vi "Strategy 5_Autotuning PID_With GUI_Modified for Testing - Copy.vi"() -> ()   [LabVIEW 2018]
doc: "This example demonstrates how to use the PID Design function to obtain PID parameters based on measured process."
uses:
  <vilib>/DAQmx/write.llb/DAQmx Write (Digital 1D Bool 1Chan 1Samp).vi
  <vilib>/DAQmx/read.llb/DAQmx Read (Analog 1D DBL NChan 1Samp).vi
  <vilib>/Instr/_visa.llb/VISA Configure Serial Port (Instr).vi
  <vilib>/DAQmx/create/channels.llb/DAQmx Create Channel (DO-Digital Output).vi
  <vilib>/DAQmx/miscellaneous.llb/DAQmx Fill In Error Info.vi
  <vilib>/addons/control/pid/pid.llb/PID Advanced (DBL).vi
  <vilib>/addons/control/pid/autopid.llb/PID Autotuning Design (Ziegler-Nichols).vi
  <vilib>/addons/control/pid/autopid.llb/PID Autotuning Design (Cohen-Coon).vi
  <vilib>/addons/control/pid/autopid.llb/PID Autotuning Design (Chien-Hrones-Reswick).vi
  <vilib>/addons/control/pid/autopid.llb/PID Autotuning Design (Internal Model Control).vi
  <vilib>/addons/control/pid/NI_PID_autopid.lvlib
  <vilib>/addons/control/pid/NI_PID_pid.lvlib
  <vilib>/ptbypt/NI_PtbyPt.lvlib
panel:
  out "Tracker 4 - X,Y,Z":cluster{"x":sgl, "y":sgl, "z":sgl}(graph)
  out "Tracker 3 - X,Y,Z":cluster{"x":sgl, "y":sgl, "z":sgl}(graph)
  out "Tracker 2 - X,Y,Z":cluster{"x":sgl, "y":sgl, "z":sgl}(graph)
  out "Tracker 1 - X,Y,Z":cluster{"x":sgl, "y":sgl, "z":sgl}(graph)
  in  "Set Point 1,5":dbl
  out "Real time Data 1,5":dbl[][](graph)
  in  "Set Point 3,4":dbl
  out "Real time Data 3,4":dbl[][](graph)
  in  "Set Point 2":dbl
  out "Real time Data 2":dbl[][](graph)
  in  "Set Point 7":dbl
  out "Real time Data 7":dbl[][](graph)
  in  "Set Point  6,8,9,10":dbl
  out "Real time Data 6,8,9,10":dbl[][](graph)
  in  "Set Point 11,12":dbl
  out "Real time Data -11,12":dbl[][](graph)
  out "error out":errorcluster {"code" format="%.0x"}
  in  "XYZAER":T1(array[cluster]) {"r" format="%1_6f"; "e" format="%1_6f"; "a" format="%1_6f"; "z" format="%1_6f"; "y" format="%1_6f"; "x" format="%1_6f"}
  out "Start Time Text":string
  out "Stop Time Text":string
  out "Elapsed Time Text":string
  out "HostFrameCount":u32
  out "Loop Iter":i32
  out "PnoData":bool
  in  "stop":bool
  out "?":bool
  in  "Muscle Control":T2(tab)=enum."M-11,12"
  out "Tuned PID gains 12":T3={"proportional gain (Kc)"=1.9838195929127882, "integral time (Ti, min)"=0.01995856284686879, "derivative time (Td, min)"=0.0} {"derivative time (Td, min)" format="%#.6g"; "integral time (Ti, min)" format="%#.6g"; "proportional gain (Kc)" format="%#.6g"}
  in  "Accept gain 12":bool
  in  "Control 12":T4(tab)
  in  "Ziegler-Nichols speed 12":u16(ring) items=["Fast", "Normal", "Slow"]
  in  "Tuning specifications 12":u16(ring) items=["Regulator - 0 %", "Regulator -  20%", "Servo - 0%", "Servo - 20%"]
  in  "Multiplicative factor 12":dbl(slide)=1.0 scale=0.01..100.0
  in  "Type of controller 12":u16(ring)=2 items=["P", "PI", "PID"]
  in  "Stop 12":bool
  in  "PID Gains 12":T3={"proportional gain (Kc)"=0.1625, "integral time (Ti, min)"=1.25, "derivative time (Td, min)"=0.0} {"derivative time (Td, min)" format="%#.6g"; "integral time (Ti, min)" format="%#.6g"; "proportional gain (Kc)" format="%#.6g"}
  in  "Autotune 12":bool
  in  "Reinitialize 12":bool
  in  "Excitation 12":dbl=0.5 format="%.2f"
  in  "Automatic 12":bool=TRUE
  in  "MV: 12":dbl(slide)=20.39115328927357 scale=-100.0..100.0
  out "PWM Output 12":bool
  in  "Median sample length 21":i32=100
  in  "INLET 1,5 ON/OFF 3":bool=TRUE
  out "Tuned PID gains 9":T3={"proportional gain (Kc)"=1.9838195929127882, "integral time (Ti, min)"=0.01995856284686879, "derivative time (Td, min)"=0.0} {"derivative time (Td, min)" format="%#.6g"; "integral time (Ti, min)" format="%#.6g"; "proportional gain (Kc)" format="%#.6g"}
  in  "Accept gain 9":bool
  in  "Type of controller 9":u16(ring)=2 items=["P", "PI", "PID"]
  in  "Excitation 9":dbl=0.5 format="%.2f"
  in  "Control 9":T4(tab)
  in  "Ziegler-Nichols speed 9":u16(ring) items=["Fast", "Normal", "Slow"]
  in  "Tuning specifications 9":u16(ring) items=["Regulator - 0 %", "Regulator -  20%", "Servo - 0%", "Servo - 20%"]
  in  "Multiplicative factor 9":dbl(slide)=1.0 scale=0.01..100.0
  in  "Stop 9":bool
  in  "PID Gains 9":T3={"proportional gain (Kc)"=0.1625, "integral time (Ti, min)"=1.25, "derivative time (Td, min)"=0.0} {"derivative time (Td, min)" format="%#.6g"; "integral time (Ti, min)" format="%#.6g"; "proportional gain (Kc)" format="%#.6g"}
  in  "Autotune 9":bool
  in  "Reinitialize 9":bool
  in  "Automatic 9":bool=TRUE
  in  "MV: 9":dbl(slide)=20.39115328927357 scale=-100.0..100.0
  out "PWM Output 9":bool
  in  "Median sample length 18":i32=100
  in  "INLET 3,4 ON/OFF 2":bool=TRUE
  out "Tuned PID gains 8":T3={"proportional gain (Kc)"=1.9838195929127882, "integral time (Ti, min)"=0.01995856284686879, "derivative time (Td, min)"=0.0} {"derivative time (Td, min)" format="%#.6g"; "integral time (Ti, min)" format="%#.6g"; "proportional gain (Kc)" format="%#.6g"}
  in  "Accept gain 8":bool
  in  "Control 8":T4(tab)
  in  "Ziegler-Nichols speed 8":u16(ring) items=["Fast", "Normal", "Slow"]
  in  "Tuning specifications 8":u16(ring) items=["Regulator - 0 %", "Regulator -  20%", "Servo - 0%", "Servo - 20%"]
  in  "Multiplicative factor 8":dbl(slide)=1.0 scale=0.01..100.0
  in  "Type of controller 8":u16(ring)=2 items=["P", "PI", "PID"]
  in  "Stop 8":bool
  in  "PID Gains 8":T3={"proportional gain (Kc)"=0.1625, "integral time (Ti, min)"=1.25, "derivative time (Td, min)"=0.0} {"derivative time (Td, min)" format="%#.6g"; "integral time (Ti, min)" format="%#.6g"; "proportional gain (Kc)" format="%#.6g"}
  in  "Autotune 8":bool
  in  "Reinitialize 8":bool
  in  "Excitation 8":dbl=0.5 format="%.2f"
  in  "Automatic 8":bool=TRUE
  in  "MV: 8":dbl(slide)=20.39115328927357 scale=-100.0..100.0
  out "PWM Output 8":bool
  in  "Median sample length 17":i32=100
  in  "INLET 2 ON/OFF 2":bool=TRUE
  out "Tuned PID gains 7":T3={"proportional gain (Kc)"=1.9838195929127882, "integral time (Ti, min)"=0.01995856284686879, "derivative time (Td, min)"=0.0} {"derivative time (Td, min)" format="%#.6g"; "integral time (Ti, min)" format="%#.6g"; "proportional gain (Kc)" format="%#.6g"}
  in  "Accept gain 7":bool
  in  "Control 7":T4(tab)
  in  "Ziegler-Nichols speed 7":u16(ring) items=["Fast", "Normal", "Slow"]
  in  "Tuning specifications 7":u16(ring) items=["Regulator - 0 %", "Regulator -  20%", "Servo - 0%", "Servo - 20%"]
  in  "Multiplicative factor 7":dbl(slide)=1.0 scale=0.01..100.0
  in  "Type of controller 7":u16(ring)=2 items=["P", "PI", "PID"]
  in  "Stop 7":bool
  in  "PID Gains 7":T3={"proportional gain (Kc)"=0.1625, "integral time (Ti, min)"=1.25, "derivative time (Td, min)"=0.0} {"derivative time (Td, min)" format="%#.6g"; "integral time (Ti, min)" format="%#.6g"; "proportional gain (Kc)" format="%#.6g"}
  in  "Autotune 7":bool
  in  "Reinitialize 7":bool
  in  "Excitation 7":dbl=0.5 format="%.2f"
  in  "Automatic 7":bool=TRUE
  in  "MV: 7":dbl(slide)=20.39115328927357 scale=-100.0..100.0
  out "PWM Output 7":bool
  in  "Median sample length 16":i32=100
  in  "INLET 7 ON/OFF 2":bool=TRUE
  out "Tuned PID gains 6":T3={"proportional gain (Kc)"=1.9838195929127882, "integral time (Ti, min)"=0.01995856284686879, "derivative time (Td, min)"=0.0} {"derivative time (Td, min)" format="%#.6g"; "integral time (Ti, min)" format="%#.6g"; "proportional gain (Kc)" format="%#.6g"}
  in  "Accept gain 6":bool
  in  "Control 6":T4(tab)
  in  "Ziegler-Nichols speed 6":u16(ring) items=["Fast", "Normal", "Slow"]
  in  "Tuning specifications 6":u16(ring) items=["Regulator - 0 %", "Regulator -  20%", "Servo - 0%", "Servo - 20%"]
  in  "Multiplicative factor 6":dbl(slide)=1.0 scale=0.01..100.0
  in  "Type of controller 6":u16(ring)=2 items=["P", "PI", "PID"]
  in  "Stop 6":bool
  in  "PID Gains 6":T3={"proportional gain (Kc)"=0.1625, "integral time (Ti, min)"=1.25, "derivative time (Td, min)"=0.0} {"derivative time (Td, min)" format="%#.6g"; "integral time (Ti, min)" format="%#.6g"; "proportional gain (Kc)" format="%#.6g"}
  in  "Autotune 6":bool
  in  "Reinitialize 6":bool
  in  "Excitation 6":dbl=0.5 format="%.2f"
  in  "Automatic 6":bool=TRUE
  in  "MV: 6":dbl(slide)=20.39115328927357 scale=-100.0..100.0
  out "PWM Output 6":bool
  in  "Median sample length 15":i32=100
  in  "INLET 6 ON/OFF 2":bool=TRUE
  in  "INLET":bool=TRUE
  out "PWM Output":bool
  in  "MV:":dbl(slide)=20.39115328927357 scale=-100.0..100.0
  in  "Median sample length":i32=100
  in  "Excitation":dbl=0.5 format="%.2f"
  in  "Type of controller":u16(ring)=2 items=["P", "PI", "PID"]
  in  "Control":T4(tab)
  in  "Ziegler-Nichols speed":u16(ring) items=["Fast", "Normal", "Slow"]
  in  "Tuning specifications":u16(ring) items=["Regulator - 0 %", "Regulator -  20%", "Servo - 0%", "Servo - 20%"]
  in  "Multiplicative factor":dbl(slide)=1.0 scale=0.01..100.0
  in  "Automatic":bool=TRUE
  in  "Reinitialize":bool
  in  "Accept gain":bool
  out "Tuned PID gains":T3={"proportional gain (Kc)"=1.9838195929127882, "integral time (Ti, min)"=0.01995856284686879, "derivative time (Td, min)"=0.0} {"derivative time (Td, min)" format="%#.6g"; "integral time (Ti, min)" format="%#.6g"; "proportional gain (Kc)" format="%#.6g"}
  in  "Autotune":bool
  in  "PID Gains":T3={"proportional gain (Kc)"=0.1625, "integral time (Ti, min)"=1.25, "derivative time (Td, min)"=0.0} {"derivative time (Td, min)" format="%#.6g"; "integral time (Ti, min)" format="%#.6g"; "proportional gain (Kc)" format="%#.6g"}
  in  "Stop":bool
  in  "M-11,12":i32=5
  in  "M-6,8,9,10":i32=5
  in  "M-7":i32=5
  in  "M-2":i32=5
  in  "M-3,4":i32=5
  in  "M-1,5":i32=5
  out "Stimulus operating point 12":dbl=20.314221540357543
  out "Response operating point 12":dbl=51.08345461694337
  out "Identified Plant Parameters 12":T5={"Plant Gain (K)"=1.7609511324977591, "Time Constant (T)"=1.9621978490901302, "Dead Time (L)"=0.22467425343567116}
  out "Control Output 12":dbl[](graph)
  out "Measurement 12":dbl[](graph)
  out "Stimulus operating point 9":dbl=20.314221540357543
  out "Response operating point 9":dbl=51.08345461694337
  out "Identified Plant Parameters 9":T5={"Plant Gain (K)"=1.7609511324977591, "Time Constant (T)"=1.9621978490901302, "Dead Time (L)"=0.22467425343567116}
  out "Control Output 9":dbl[](graph)
  out "Measurement 9":dbl[](graph)
  out "Identified Plant Parameters":T5={"Plant Gain (K)"=1.7609511324977591, "Time Constant (T)"=1.9621978490901302, "Dead Time (L)"=0.22467425343567116}
  out "Control Output":dbl[](graph)
  out "Measurement":dbl[](graph)
  out "Stimulus operating point":dbl=20.314221540357543
  out "Response operating point":dbl=51.08345461694337
  out "Stimulus operating point 6":dbl=20.314221540357543
  out "Response operating point 6":dbl=51.08345461694337
  out "Identified Plant Parameters 6":T5={"Plant Gain (K)"=1.7609511324977591, "Time Constant (T)"=1.9621978490901302, "Dead Time (L)"=0.22467425343567116}
  out "Control Output 6":dbl[](graph)
  out "Measurement 6":dbl[](graph)
  out "Stimulus operating point 7":dbl=20.314221540357543
  out "Response operating point 7":dbl=51.08345461694337
  out "Identified Plant Parameters 7":T5={"Plant Gain (K)"=1.7609511324977591, "Time Constant (T)"=1.9621978490901302, "Dead Time (L)"=0.22467425343567116}
  out "Control Output 7":dbl[](graph)
  out "Measurement 7":dbl[](graph)
  out "Stimulus operating point 8":dbl=20.314221540357543
  out "Response operating point 8":dbl=51.08345461694337
  out "Identified Plant Parameters 8":T5={"Plant Gain (K)"=1.7609511324977591, "Time Constant (T)"=1.9621978490901302, "Dead Time (L)"=0.22467425343567116}
  out "Control Output 8":dbl[](graph)
  out "Measurement 8":dbl[](graph)
  out "Connected":bool
  out "Running":bool
  out "Position Sensor Data":cluster{dbl, "x":sgl}[](graph)
  out "Sensor Raw Value 2":i32
  in  "COM Port-Sensor 2":refnum<visa-resource-name>="COM5"
  in  "upper/lower infle":enum32{"Page 1", "Page 2"}(tab)
  out "Force in Kilograms":dbl(graph)
  out "Force in Newtons":dbl(graph)
  in  "lower/upper infle":enum32{"Page 1", "Page 2"}(tab)
  out "Force in Newtons 2":dbl(graph)
  out "Force in Kilograms 2":dbl(graph)
  in  "COM Port-Sensor 1":refnum<visa-resource-name>="COM4"
  out "Sensor Raw Value":i32
  in  "Tab Control":T6(tab)
  in  "Instructions":string="Overview: This example demonstrates how to use the PID Autotuning Design to obtain PID parameters based on setpoint and process variable collected in another loop.\nInstructions:\n1. Run the VI and wait until the process variable (PV) reaches near setpoint (SP).\n2.  In the PID Autotuning Design section, select the type of algorithm, type of controller and excitation amplitude for the 'open loop step response'. Then, click Autotune to start the process. Select the Identified Plant Parameter tab and see the results from the identification.\n3.  When the tuned PID gains do not change anymore, the identification is done and you have the option to accept by clicking Accept gain, which will transfer the new gain to PID Gains.\n4. Click the Autotune button again to go back to the automatic control state. You can try different options and repeat this process.\n5. Click Stop to stop the VI.\n"
  # "Pressure Alarm"
  # "Force Sensor Data"
  # "Position Sensor Data"
  # "PID Controller"
  # "PID Autotuning Design"
  # "No additional parameters"
  # "PID Controller"
  # "PID Autotuning Design"
  # "No additional parameters"
  # "PID Controller"
  # "PID Autotuning Design"
  # "No additional parameters"
  # "PID Controller"
  # "PID Autotuning Design"
  # "No additional parameters"
  # "PID Controller"
  # "PID Autotuning Design"
  # "No additional parameters"
  # "Muscle Control"
  # "PID Controller"
  # "PID Autotuning Design"
  # "No additional parameters"
  # "Pressure Cut Off to trigger the alarm"
  # "M-11,12"
  # "M-3,4"
  # "M-1,5"
  # "M-6,8,9,10"
  # "M-7"
  # "M-2"
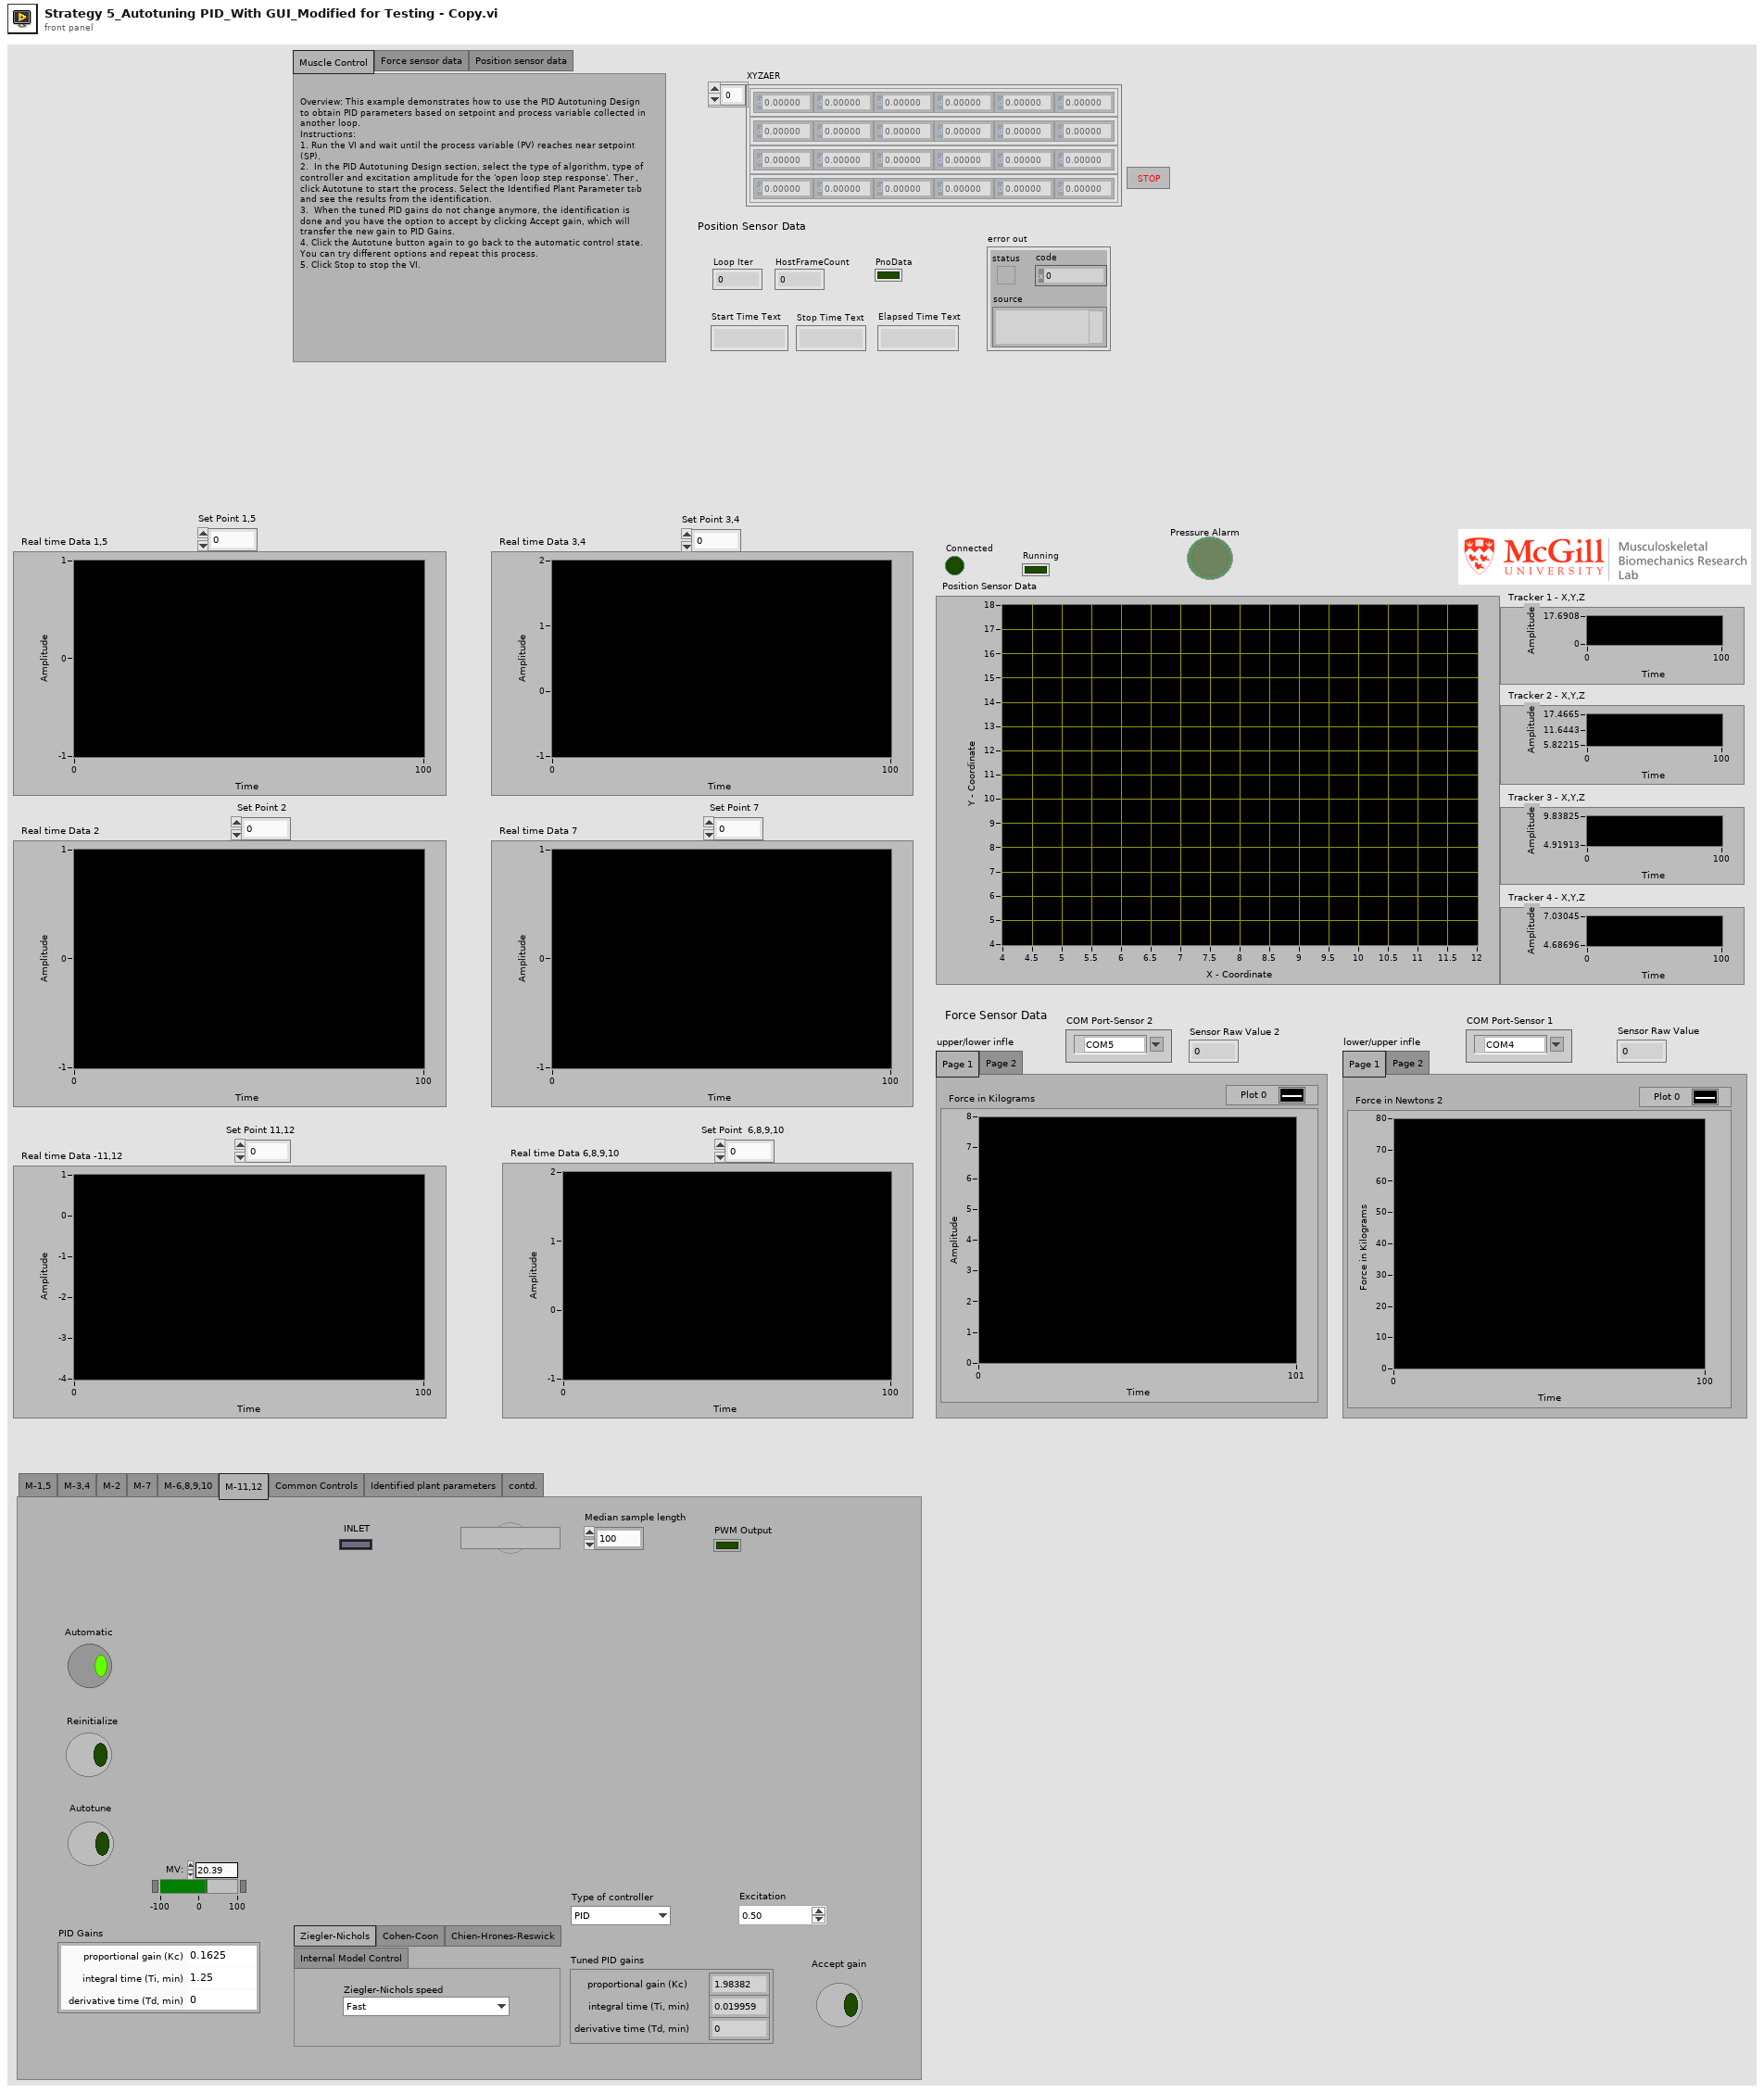
[diagram p1: front panel]
types:
  T1 = cluster{"x":sgl, "y":sgl, "z":sgl, "a":sgl, "e":sgl, "r":sgl}[]
  T2 = enum32{"M-1,5", "M-3,4", "M-2", "M-7", "M-6,8,9,10", "M-11,12", "Common Controls", "Identified plant parameters", "contd."}
  T3 = cluster{"proportional gain (Kc)":dbl, "integral time (Ti, min)":dbl, "derivative time (Td, min)":dbl}
  T4 = enum32{"Ziegler-Nichols", "Cohen-Coon", "Chien-Hrones-Reswick", "Internal Model Control"}
  T5 = cluster{"Plant Gain (K)":dbl, "Time Constant (T)":dbl, "Dead Time (L)":dbl}
  T6 = enum32{"Muscle Control", "Force sensor data", "Position sensor data"}
  T7 = cluster{"static gain":dbl, "lag (s)":dbl, "deadtime (s)":dbl, "load":dbl, "deadband":dbl, "sensor noise":dbl, "initial PV":dbl, "plant noise":dbl}
  T8 = cluster{"x":sgl, "y":sgl, "z":sgl, "a":sgl, "e":sgl, "r":sgl}
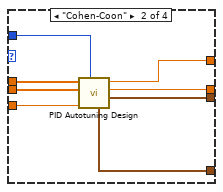
[diagram p2: hidden frame]
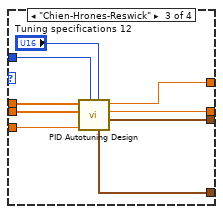
[diagram p3: hidden frame]
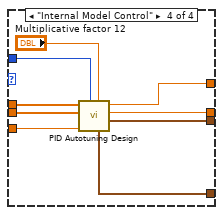
[diagram p4: hidden frame]
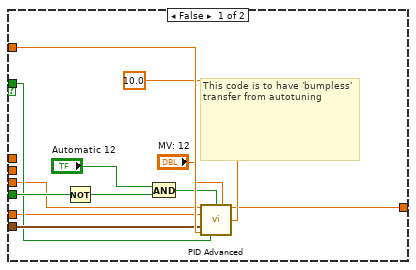
[diagram p6: hidden frame]
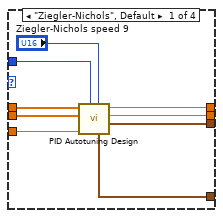
[diagram p7: hidden frame]
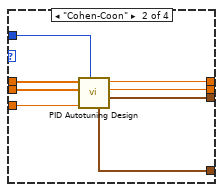
[diagram p8: hidden frame]
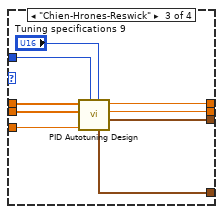
[diagram p9: hidden frame]
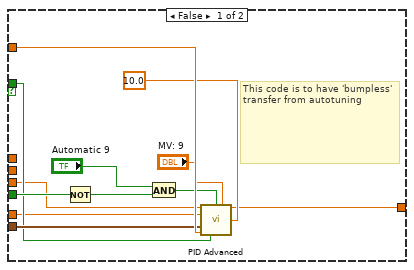
[diagram p11: hidden frame]
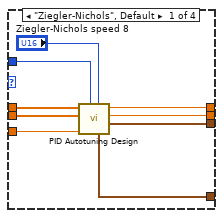
[diagram p12: hidden frame]
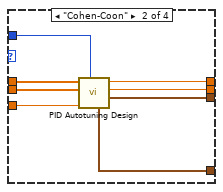
[diagram p13: hidden frame]
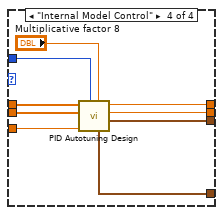
[diagram p14: hidden frame]
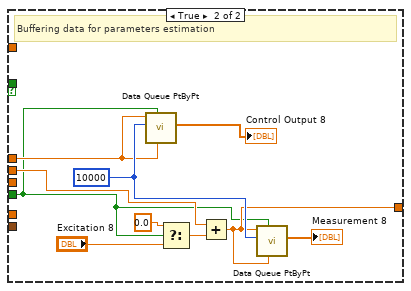
[diagram p16: hidden frame]
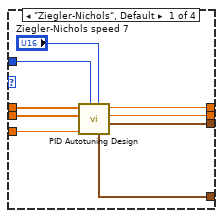
[diagram p17: hidden frame]
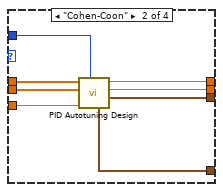
[diagram p18: hidden frame]
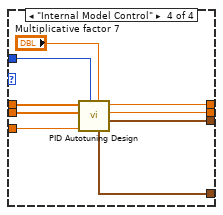
[diagram p19: hidden frame]
diagram:
  w19 = 0.0 ("output")
  w22 = FALSE ("Stop")
  w25 = 0.0 ("output")
  w28 = FALSE ("Stop")
  w31 = 0.0 ("output")
  w34 = FALSE ("Stop")
  w37 = 0.0 ("output")
  w40 = FALSE ("Stop")
  w43 = 0.0 ("output")
  w46 = FALSE ("Stop")
  w51 = 2400  # BufferFrameCount
  w85 = 0.0 ("output")
  w88 = FALSE ("Stop")
  # "Muscle-1,5 PID CONTROL LOOP (Auto Tuning)"
  # "Muscle-3,4 PID CONTROL LOOP (Auto Tuning)"
  # "Muscle-2 PID CONTROL LOOP (Auto Tuning)"
  # "Muscle-7 PID CONTROL LOOP (Auto Tuning)"
  # "Muscle-6,8,9,10 PID CONTROL LOOP (Auto Tuning)"
  # "Muscle-11,12 PID CONTROL LOOP (Auto Tuning)"
  # "FORCE SENSOR CONTROL LOOP"
  # "POSITION SENSOR CONTROL LOOP"
  # "Pressure Alarm"
  # "8. Close Tracker connection."
  # "3. Query Max num sensors supported by the tracker."
  # "4. Allocate raw buffer to hold 2400 frames of data."
  # "5. Start Continuous mode."
  # "7. Stop Continuous mode."
  # "6. Start the loop. Loop exits when Stop Button is hit."
  n1 = Obtain Queue(element data type=0.0) -> (queue out=w12:refnum<queue>)  [unwired: 4 in, 2 out]
  n2 = while {
    shift-left: 0.0 ("Plant Output") -> [w204]
    shift-right: [w199] -> _
    tunnel: w46 -> [_]
    shift-right: [w185] -> _
    shift-left: 0.01 -> [w183]
    shift-right: [w158] -> _
    shift-left: TRUE -> [w182]
    shift-right: [w160] -> _
    shift-left: w43 -> [w181]
    shift-right: [w184] -> _
    shift-left: w43 -> [w180]
    tunnel: [w155] -> w42
    tunnel: [w142] -> w2
    tunnel: w12 -> [w140]
    stop <- "Stop 6" stop-if-true
    w93 = 1 items=["one channel for each line", "one channel for all lines"] ("line grouping")
    w101 = 1 items=["one channel for each line", "one channel for all lines"] ("line grouping")
    w109 = 1 items=["one channel for each line", "one channel for all lines"] ("line grouping")
    w117 = 1 items=["one channel for each line", "one channel for all lines"] ("line grouping")
    w125 = 1 items=["one channel for each line", "one channel for all lines"] ("line grouping")
    w133 = 1 items=["one channel for each line", "one channel for all lines"] ("line grouping")
    w146 = 1 items=["one channel for each line", "one channel for all lines"] ("line grouping")
    w155 = 0.05 ("Sampling Time dt (s)")
    w163 = 1 items=["one channel for each line", "one channel for all lines"] ("line grouping")
    w171 = 0.5 ("x")
    w198 = T7 {"static gain"=2.5, "lag (s)"=2.5, "deadtime (s)"=0.01, "load"=0.0, "deadband"=0.0, "sensor noise"=0.0, "initial PV"=30.0, "plant noise"=0.0}  # Process parameters
    w200 = FALSE  # Integrator ?
    # "Inlet 11"
    # "Exhaust 10"
    # "Inlet 11"
    # "Exhaust 9"
    # "Inlet 11"
    # "Exhaust 8"
    # "C."
    # "Inlet 11"
    # "Exhaust 6"
    # "B."
    # "A."
    # "A.Output to PWM Logic \nB. Simulated Plant\nC. Draw Chart"
    # "Main PID Loop Control"
    n3 = Dequeue Element(queue=w140) -> (element=w141:dbl)  [unwired: 2 in, 3 out]
    n4 = Multiply(x=w155, y=1000.0) -> (x*y=w197:dbl)
    n5 = Not(x="Autotune 6") -> (.not. x?=w201:bool)
    n6 = feedback #1() -> (w206:bool)  [unwired: 1 in]
    n7 = feedback-in #1("Autotune 6") -> ()
    n8 = Wait Until Next ms Multiple(millisecond multiple=w197) -> ()  [unwired: 1 out]
    n9 = Exclusive Or(1:w206, 2:"Autotune 6") -> (0:w205:bool)
    n10 = feedback #2() -> (w203:dbl)  [unwired: 1 in]
    n11 = Multiply(x=w141, y=-1000.0) -> (x*y=w187:dbl)
    n12 = call <vilib>:"Median PtByPt.vi"("sample length"="Median sample length 15", "x"=w187) -> ("median"=w186:dbl)  [unwired: 2 in, 1 out]
    n13 = Square(x=w186) -> (x^2=w194:dbl)
    n14 = Multiply(x=w186, y=16.572) -> (x*y=w190:dbl)
    n15 = Multiply(x=w194, y=-0.06) -> (x*y=w191:dbl)
    n16 = Add(x=w190, y=w191) -> (x+y=w189:dbl)
    n17 = Add(x=-1011.3, y=w189) -> (x+y=w153:dbl)
    n18 = case shown="False" "Autotune 6" {
      tunnel: w155 -> [w221 _]
      tunnel: [w210 w226] -> w160
      tunnel: w204 -> [_ w225]
      tunnel: "PID Gains 6" -> [w220 _]
      tunnel: "Reinitialize 6" -> [w217 _]
      tunnel: w205 -> [w219 w224]
      tunnel: w203 -> [_ w228]
      tunnel: w153 -> [w213 _]
      tunnel: "Set Point  6,8,9,10" -> [w212 _]
      frame False {
        # "This code is to have 'bumpless' transfer from autotuning"
        n19 = Not(x=w219) -> (.not. x?=w216:bool)
        n20 = And(x="Automatic 6", y=w216) -> (x .and. y?=w218:bool)
        n21 = call-poly <vilib>:"PID Advanced.vi"("setpoint"=w212, "auto? (T)"=w218, "manual control"="MV: 6", "process variable"=w213, "alpha"=10.0, "PID gains"=w220, "dt (s)"=w221, "reinitialize? (F)"=w217) -> ("output"=w210:dbl)  [unwired: 6 in, 1 out]
      }
      frame True {
        w231 = 10000 ("sample length")
        # "Buffering data for parameters estimation"
        n22 = call <vilib>:"Data Queue PtByPt.vi"("initial queue element"=w225, "initialize"=w224, "sample length"=w231, "input data point"=w225) -> ("Current Queue"=→"Control Output 6":dbl[])  [unwired: 3 in, 4 out]
        n23 = Select(t=0.0, s=w224, f="Excitation 6") -> (s? t:f=w229:dbl)
        n24 = Add(x=w228, y=w229) -> (x+y=w226:dbl)
        n25 = call <vilib>:"Data Queue PtByPt.vi"("initial queue element"=w226, "initialize"=w224, "sample length"=w231, "input data point"=w226) -> ("Current Queue"=→"Measurement 6":dbl[])  [unwired: 3 in, 4 out]
      }
    }
    n26 = feedback-in #2(w160, w201) -> ()
    n27 = Greater?(x=w153, y="M-6,8,9,10") -> (0:w142:bool)
    n28 = Add(x=w183, y=w171) -> (x+y=w172:dbl)
    n29 = Subtract(x=w183, y=w171) -> (x-y=w170:dbl)
    n30 = Equal?(x=w181, y=w160) -> (x = y?=w178:bool)
    n31 = Greater?(x=w160, y=w181) -> (0:w177:bool)
    n32 = Select(t=w182, s=w178, f=w177) -> (s? t:f=w158:bool)
    "PWM Output 6" <- w158
    n33 = call "Plant System.vi"("Integrator ?"=w200, "Plant Input"=w160, "dt (s)"=w155, "process parameters"=w198) -> ("Plant Output"=w199:dbl)  [unwired: 11 in]
    n34 = Increment(x="Set Point  6,8,9,10") -> (x+1=w176:dbl)
    n35 = Decrement(x="Set Point  6,8,9,10") -> (x-1=w175:dbl)
    n36 = Select(t=w172, s=w158, f=w170) -> (s? t:f=w185:dbl)
    n37 = call-poly <vilib>:"DAQmx Create Virtual Channel.vi"("lines"=tag "cDAQ1Mod1/port0/line3", "line grouping"=w117) -> ("task out"=w119:refnum<k21>, "error out"=w118:errorcluster)  [unwired: 12 in]
    n38 = call-poly <vilib>:"DAQmx Create Virtual Channel.vi"("lines"=tag "cDAQ1Mod2/port0/line3", "line grouping"=w109) -> ("task out"=w111:refnum<k21>, "error out"=w110:errorcluster)  [unwired: 12 in]
    n39 = Select(t=w176, s=w158, f=w175) -> (s? t:f=w174:dbl)
    n40 = Not(x=w158) -> (.not. x?=w157:bool)
    n41 = call-poly <vilib>:"DAQmx Create Virtual Channel.vi"("lines"=tag "cDAQ1Mod1/port0/line4", "line grouping"=w163) -> ("task out"=w165:refnum<k21>, "error out"=w164:errorcluster)  [unwired: 12 in]
    n42 = call-poly <vilib>:"DAQmx Create Virtual Channel.vi"("lines"=tag "cDAQ1Mod2/port0/line4", "line grouping"=w146) -> ("task out"=w148:refnum<k21>, "error out"=w147:errorcluster)  [unwired: 12 in]
    n43 = Build Array(w153, "Set Point  6,8,9,10", w174) -> (w173:dbl[])
    n44 = Initialize Array("INLET 6 ON/OFF 2", 1 ("dimension size")) -> (w90:bool[])
    n45 = Initialize Array(w157, 1 ("dimension size")) -> (w91:bool[])
    n46 = local write "MV: 6"(w160) -> ()
    n47 = Add(x=w180, y=w183) -> (x+y=w184:dbl)
    n48 = Build Array(w173) -> (→"Real time Data 6,8,9,10":dbl[][])
    n49 = call-poly <vilib>:"DAQmx Write.vi"("task/channels in"=w119, "auto start"=TRUE, "data"=w91, "error in"=w118) -> ("task out"=w121:refnum<k21>, "error out"=w122:errorcluster)  [unwired: 9 in, 1 out]
    n50 = call-poly <vilib>:"DAQmx Write.vi"("task/channels in"=w111, "auto start"=TRUE, "data"=w90, "error in"=w110) -> ("task out"=w113:refnum<k21>, "error out"=w114:errorcluster)  [unwired: 9 in, 1 out]
    n51 = call-poly <vilib>:"DAQmx Write.vi"("task/channels in"=w165, "auto start"=TRUE, "data"=w91, "error in"=w164) -> ("task out"=w167:refnum<k21>, "error out"=w168:errorcluster)  [unwired: 9 in, 1 out]
    n52 = call-poly <vilib>:"DAQmx Write.vi"("task/channels in"=w148, "auto start"=TRUE, "data"=w90, "error in"=w147) -> ("task out"=w150:refnum<k21>, "error out"=w151:errorcluster)  [unwired: 9 in, 1 out]
    n53 = call <vilib>:"DAQmx Clear Task.vi"("task in"=w121, "error in"=w122) -> ("error out"=w116:errorcluster)  [unwired: 13 in]
    n54 = call <vilib>:"DAQmx Clear Task.vi"("task in"=w113, "error in"=w114) -> ("error out"=w108:errorcluster)  [unwired: 13 in]
    n55 = call <vilib>:"DAQmx Clear Task.vi"("task in"=w167, "error in"=w168) -> ("error out"=w162:errorcluster)  [unwired: 13 in]
    n56 = call <vilib>:"DAQmx Clear Task.vi"("task in"=w150, "error in"=w151) -> ("error out"=w145:errorcluster)  [unwired: 13 in]
    n57 = call <vilib>:"Simple Error Handler.vi"("error in (no error)"=w116) -> ()  [unwired: 4 in, 5 out]
    n58 = call <vilib>:"Simple Error Handler.vi"("error in (no error)"=w108) -> ()  [unwired: 4 in, 5 out]
    n59 = call <vilib>:"Simple Error Handler.vi"("error in (no error)"=w162) -> ()  [unwired: 4 in, 5 out]
    n60 = call <vilib>:"Simple Error Handler.vi"("error in (no error)"=w145) -> ()  [unwired: 4 in, 5 out]
    n61 = call-poly <vilib>:"DAQmx Create Virtual Channel.vi"("lines"=tag "cDAQ1Mod8/port0/line6", "line grouping"=w101) -> ("task out"=w103:refnum<k21>, "error out"=w102:errorcluster)  [unwired: 12 in]
    n62 = call-poly <vilib>:"DAQmx Create Virtual Channel.vi"("lines"=tag "cDAQ1Mod7/port0/line5", "line grouping"=w93) -> ("task out"=w95:refnum<k21>, "error out"=w94:errorcluster)  [unwired: 12 in]
    n63 = call-poly <vilib>:"DAQmx Create Virtual Channel.vi"("lines"=tag "cDAQ1Mod8/port0/line3", "line grouping"=w133) -> ("task out"=w135:refnum<k21>, "error out"=w134:errorcluster)  [unwired: 12 in]
    n64 = call-poly <vilib>:"DAQmx Create Virtual Channel.vi"("lines"=tag "cDAQ1Mod7/port0/line2", "line grouping"=w125) -> ("task out"=w127:refnum<k21>, "error out"=w126:errorcluster)  [unwired: 12 in]
    n65 = call-poly <vilib>:"DAQmx Write.vi"("task/channels in"=w103, "auto start"=TRUE, "data"=w91, "error in"=w102) -> ("task out"=w105:refnum<k21>, "error out"=w106:errorcluster)  [unwired: 9 in, 1 out]
    n66 = call-poly <vilib>:"DAQmx Write.vi"("task/channels in"=w95, "auto start"=TRUE, "data"=w90, "error in"=w94) -> ("task out"=w97:refnum<k21>, "error out"=w98:errorcluster)  [unwired: 9 in, 1 out]
    n67 = call-poly <vilib>:"DAQmx Write.vi"("task/channels in"=w135, "auto start"=TRUE, "data"=w91, "error in"=w134) -> ("task out"=w137:refnum<k21>, "error out"=w138:errorcluster)  [unwired: 9 in, 1 out]
    n68 = call-poly <vilib>:"DAQmx Write.vi"("task/channels in"=w127, "auto start"=TRUE, "data"=w90, "error in"=w126) -> ("task out"=w129:refnum<k21>, "error out"=w130:errorcluster)  [unwired: 9 in, 1 out]
    n69 = call <vilib>:"DAQmx Clear Task.vi"("task in"=w105, "error in"=w106) -> ("error out"=w100:errorcluster)  [unwired: 13 in]
    n70 = call <vilib>:"DAQmx Clear Task.vi"("task in"=w97, "error in"=w98) -> ("error out"=w92:errorcluster)  [unwired: 13 in]
    n71 = call <vilib>:"DAQmx Clear Task.vi"("task in"=w137, "error in"=w138) -> ("error out"=w132:errorcluster)  [unwired: 13 in]
    n72 = call <vilib>:"DAQmx Clear Task.vi"("task in"=w129, "error in"=w130) -> ("error out"=w124:errorcluster)  [unwired: 13 in]
    n73 = call <vilib>:"Simple Error Handler.vi"("error in (no error)"=w100) -> ()  [unwired: 4 in, 5 out]
    n74 = call <vilib>:"Simple Error Handler.vi"("error in (no error)"=w92) -> ()  [unwired: 4 in, 5 out]
    n75 = call <vilib>:"Simple Error Handler.vi"("error in (no error)"=w132) -> ()  [unwired: 4 in, 5 out]
    n76 = call <vilib>:"Simple Error Handler.vi"("error in (no error)"=w124) -> ()  [unwired: 4 in, 5 out]
  }
  n77 = local write "Stop 6"(w46) -> ()
  n78 = while {
    tunnel: w46 -> [_]
    tunnel: w42 -> [w235]
    stop <- w245 stop-if-true
    # "If dT and deadtime have similar values, the identification could evaluate deadtime as zero and this generates proportional gain equal to Inf. This code avoid gain changes in this situations."
    # "Autotuning Loop"
    n79 = local read "Control Output 6"() -> (w247:dbl[])
    n80 = local read "Measurement 6"() -> (w246:dbl[])
    n81 = case shown="\"Chien-Hrones-Reswick\"" "Control 6" {
      tunnel: w247 -> [w256 w264 w273 w282]
      tunnel: w246 -> [w255 w263 w272 w281]
      tunnel: [w254 w262 w271 w280] -> w234
      tunnel: [w253 w261 w270 w279] -> w233
      tunnel: w235 -> [w252 w260 w269 w278]
      tunnel: [w251 w259 w268 w277] -> w232
      tunnel: [w250 w258 w267 w276] -> w237
      tunnel: "Type of controller 6" -> [w249 w257 w266 w275]
      frame "Ziegler-Nichols", Default {
        n82 = call-poly <vilib>:"PID Autotuning Design.vi"("Ziegler-Nichols Speed"="Ziegler-Nichols speed 6", "Type of Controller"=w249, "dt (s)"=w252, "Response signal"=w255, "Stimulus signal"=w256) -> ("PID gains"=w250:T3, "response operating point"=w253:dbl, "stimulus operating point"=w254:dbl, "Plant Parameters"=w251:T5)  [unwired: 3 in]
      }
      frame "Cohen-Coon" {
        n83 = call-poly <vilib>:"PID Autotuning Design.vi"("Type of Controller"=w257, "dt (s)"=w260, "Response signal"=w263, "Stimulus signal"=w264) -> ("PID gains"=w258:T3, "response offset"=w261:dbl, "stimulus offset"=w262:dbl, "Plant Parameters"=w259:T5)  [unwired: 4 in]
      }
      frame "Chien-Hrones-Reswick" {
        n84 = call-poly <vilib>:"PID Autotuning Design.vi"("Tuning specifications"="Tuning specifications 6", "Type of Controller"=w266, "dt (s)"=w269, "Response signal"=w272, "Stimulus signal"=w273) -> ("PID gains"=w267:T3, "response offset"=w270:dbl, "stimulus offset"=w271:dbl, "Plant Parameters"=w268:T5)  [unwired: 3 in]
      }
      frame "Internal Model Control" {
        n85 = call-poly <vilib>:"PID Autotuning Design.vi"("Desired Time Constant (tau_c)"="Multiplicative factor 6", "Type of Controller"=w275, "dt (s)"=w278, "Response signal"=w281, "Stimulus signal"=w282) -> ("PID gains"=w276:T3, "response offset"=w279:dbl, "stimulus offset"=w280:dbl, "Plant Parameters"=w277:T5)  [unwired: 3 in]
      }
    }
    "Stimulus operating point 6" <- w234
    "Response operating point 6" <- w233
    "Identified Plant Parameters 6" <- w232
    n86 = Unbundle(w237) -> ("proportional gain (Kc)"=w240:dbl)  [unwired: 2 out]
    n87 = Equal?(x=w240, y=inf) -> (x = y?=w239:bool)
    n88 = feedback #3() -> (w238:T3)  [unwired: 1 in]
    n89 = Select(t=w238, s=w239, f=w237) -> (s? t:f=w236:T3)
    "Tuned PID gains 6" <- w236
    n90 = feedback-in #3(w236) -> ()
    n91 = case shown="True" "Accept gain 6" {
      tunnel: w236 -> [_ w283]
      frame False {
      }
      frame True {
        n92 = local write "PID Gains 6"(w283) -> ()
      }
    }
    n93 = local read "Stop 6"() -> (w245:bool)
  }
  n94 = local write "Stop"(w88) -> ()
  n95 = call-poly "VISA Configure Serial Port"("VISA resource name"="COM Port-Sensor 1") -> ("VISA resource name out"=w79:refnum<visa-resource-name>, "error out"=w78:errorcluster)  [unwired: 9 in, 4 out]
  n96 = call-poly "VISA Configure Serial Port"("VISA resource name"="COM Port-Sensor 2") -> ("VISA resource name out"=w74:refnum<visa-resource-name>, "error out"=w73:errorcluster)  [unwired: 9 in, 4 out]
  n97 = while {
    shift-right: [w291] -> w80
    shift-left: w79 -> [w287]
    tunnel: w78 -> [w286]
    tunnel: [w288] -> w81
    stop <- w289 stop-if-true
    # "Serial Read Loop"
    n98 = case shown="True" TRUE {
      tunnel: [w303 w307] -> w291
      tunnel: w287 -> [w305 w307]
      tunnel: [w302 w306] -> w288
      tunnel: w286 -> [w304 w306]
      frame True {
        n99 = VISA Read(VISA resource name=w305, byte count=u32 1000, error in (no error)=w304) -> (VISA resource name out=w303:refnum<visa-resource-name>, read buffer=w300:string, error out=w302:errorcluster)  [unwired: 1 out]
        n100 = Decimal String To Number(string=w300) -> (number=w298:i32)  [unwired: 2 in, 1 out]
        "Sensor Raw Value" <- w298
        n101 = call <vilib>:"Median PtByPt.vi"("sample length"=20, "x"=w298) -> ("median"=w296:dbl)  [unwired: 2 in, 1 out]
        n102 = To Double Precision Float(number=w296) -> (double precision float=w292:dbl)
        n103 = Multiply(x=w292, y=0.0292) -> (x*y=w295:dbl)
        "Force in Kilograms 2" <- w295
        n104 = Multiply(x=w295, y=9.81) -> (x*y=→"Force in Newtons 2":dbl)
      }
      frame False {
      }
    }
    n105 = Wait (ms)(milliseconds to wait=u32 5) -> ()  [unwired: 1 out]
    n106 = Or(x=w288, y=FALSE) -> (x .or. y?=w289:bool)
  }
  n107 = while {
    shift-right: [w315] -> w48
    shift-left: w74 -> [w311]
    tunnel: w73 -> [w310]
    tunnel: [w312] -> w75
    stop <- w313 stop-if-true
    # "Serial Read Loop"
    n108 = case shown="True" TRUE {
      tunnel: [w327 w331] -> w315
      tunnel: w311 -> [w329 w331]
      tunnel: [w326 w330] -> w312
      tunnel: w310 -> [w328 w330]
      frame True {
        n109 = VISA Read(VISA resource name=w329, byte count=u32 1000, error in (no error)=w328) -> (VISA resource name out=w327:refnum<visa-resource-name>, read buffer=w324:string, error out=w326:errorcluster)  [unwired: 1 out]
        n110 = Decimal String To Number(string=w324) -> (number=w320:i32)  [unwired: 2 in, 1 out]
        "Sensor Raw Value 2" <- w320
        n111 = call <vilib>:"Median PtByPt.vi"("sample length"=20, "x"=w320) -> ("median"=w321:dbl)  [unwired: 2 in, 1 out]
        n112 = To Double Precision Float(number=w321) -> (double precision float=w317:dbl)
        n113 = Multiply(x=w317, y=0.0238) -> (x*y=w316:dbl)
        "Force in Kilograms" <- w316
        n114 = Multiply(x=w316, y=9.81) -> (x*y=→"Force in Newtons":dbl)
      }
      frame False {
      }
    }
    n115 = Or(x=w312, y=FALSE) -> (x .or. y?=w313:bool)
    n116 = Wait (ms)(milliseconds to wait=u32 5) -> ()  [unwired: 1 out]
  }
  n117 = VISA Close(VISA resource name=w80, error in (no error)=w81) -> (error out=w82:errorcluster)
  n118 = call <vilib>:"Simple Error Handler.vi"("error in (no error)"=w82) -> ()  [unwired: 1 in, 8 out]
  n119 = VISA Close(VISA resource name=w48, error in (no error)=w75) -> (error out=w76:errorcluster)
  n120 = call <vilib>:"Simple Error Handler.vi"("error in (no error)"=w76) -> ()  [unwired: 1 in, 8 out]
  n121 = stacked-sequence {
    tunnel: [_ w337] -> w55
    tunnel: [_ w336] -> w54
    frame #0 {
      w332 = 0
      w333 = FALSE
      w334 = ""
      # "Initialize Indicators"
      "Connected" <- w333
      "Start Time Text" <- w334
      "Stop Time Text" <- w334
      "Elapsed Time Text" <- w334
      "HostFrameCount" <- w332
      "Running" <- w333
      "Loop Iter" <- w332
      "PnoData" <- w333
    }
    frame #1 {
      # "Connect To Tracker"
      # "2. Initialize Tracker Connection"
      n122 = call <instrlib>:"PDI initialize.vi"() -> ("error out"=w336:errorcluster, "Connected"=w335:bool, "pDev"=w337:u32)  [unwired: 1 in, 4 out]
      n123 = local write "Connected"(w335) -> ()
    }
  }
  n124 = while {
    stop <- FALSE stop-if-true
    # "TRACKER 4"
    # "TRACKER 3"
    # "TRACKER 2"
    # "TRACKER 1"
    n125 = Index Array(array="XYZAER", index #1=0 ("index"), index #2=1 ("index"), index #3=2 ("index"), index #4=3 ("index")) -> (element #1=w370:T8, element #2=w369:T8, element #3=w368:T8, element #4=w367:T8)
    n126 = Unbundle By Name(w370) -> ("x"=w353:sgl, "y"=w352:sgl, "z"=w351:sgl)
    n127 = Unbundle By Name(w369) -> ("x"=w350:sgl, "y"=w349:sgl, "z"=w348:sgl)
    n128 = Multiply(x=w352, y=sgl -1.0) -> (x*y=w361:sgl)
    n129 = Multiply(x=w349, y=-1.0) -> (x*y=w360:dbl)
    n130 = Bundle(w360, "x"=w350) -> (w356:cluster{dbl, "x":sgl})  [unwired: 1 in]
    n131 = Bundle(w361, "x"=w353) -> (w357:cluster{sgl, "x":sgl})  [unwired: 1 in]
    n132 = Unbundle By Name(w368) -> ("x"=w347:sgl, "y"=w346:sgl, "z"=w345:sgl)
    n133 = Unbundle By Name(w367) -> ("x"=w344:sgl, "y"=w343:sgl, "z"=w342:sgl)
    n134 = Multiply(x=w346, y=-1.0) -> (x*y=w359:dbl)
    n135 = Multiply(x=w343, y=-1.0) -> (x*y=w358:dbl)
    n136 = Bundle(w359, "x"=w347) -> (w355:cluster{dbl, "x":sgl})  [unwired: 1 in]
    n137 = Bundle(w358, "x"=w344) -> (w354:cluster{dbl, "x":sgl})  [unwired: 1 in]
    n138 = Build Array(w357, w356, w355, w354) -> (→"Position Sensor Data":cluster{dbl, "x":sgl}[])
    n139 = Bundle("x"=w350, "y"=w349, "z"=w348) -> (→"Tracker 2 - X,Y,Z":cluster{"x":sgl, "y":sgl, "z":sgl})  [unwired: 1 in]
    n140 = Bundle("x"=w353, "y"=w352, "z"=w351) -> (→"Tracker 1 - X,Y,Z":cluster{"x":sgl, "y":sgl, "z":sgl})  [unwired: 1 in]
    n141 = Bundle("x"=w347, "y"=w346, "z"=w345) -> (→"Tracker 3 - X,Y,Z":cluster{"x":sgl, "y":sgl, "z":sgl})  [unwired: 1 in]
    n142 = Bundle("x"=w344, "y"=w343, "z"=w342) -> (→"Tracker 4 - X,Y,Z":cluster{"x":sgl, "y":sgl, "z":sgl})  [unwired: 1 in]
  }
  n143 = call <instrlib>:"PDI util stationcount.vi"("error in (no error)"=w54, "pDev"=w55) -> ("error out"=w53:errorcluster, "dup pDev"=w52:u32, "MaxCount"=w50:i32)  [unwired: 7 out]
  n144 = call <instrlib>:"PDI config setbuffer.vi"("error in (no error)"=w53, "Max sensors"=w50, "FrameCount"=w51, "pDev"=w52) -> ("error out"=w62:errorcluster, "dup pDev"=w63:u32)  [unwired: 6 out]
  n145 = flat-sequence {
    tunnel: w68 -> [_]
    tunnel: [w377] -> w64
    frame #0 {
      # "Get Start Time"
      n146 = Get Date/Time In Seconds() -> (seconds since 1Jan1904=w378:timestamp)
      n147 = Format Date/Time String(seconds (now)=w378) -> (date/time string=w379:string)  [unwired: 2 out]
      n148 = local write "Start Time Text"(w379) -> ()
      n149 = To Double Precision Float(number=w378) -> (double precision float=w377:dbl)
    }
  }
  n150 = call <instrlib>:"PDI action startcont.vi"("error in (no error)"=w62, "pDev"=w63) -> ("error out"=w69:errorcluster, "Running"=w61:bool, "dup pDev"=w68:u32)  [unwired: 7 out]
  n151 = control-ref of="HostFrameCount"() -> (w59:refnum<vi>)
  n152 = local write "Running"(w61) -> ()
  n153 = Obtain Queue(element data type=0.0) -> (queue out=w8:refnum<queue>)  [unwired: 4 in, 2 out]
  n154 = while {
    shift-left: 0.0 ("Plant Output") -> [w462]
    shift-right: [w457] -> _
    tunnel: w28 -> [_]
    shift-right: [w443] -> _
    shift-left: 0.01 -> [w441]
    shift-right: [w416] -> _
    shift-left: TRUE -> [w440]
    shift-right: [w418] -> _
    shift-left: w25 -> [w439]
    shift-right: [w442] -> _
    shift-left: w25 -> [w438]
    tunnel: [w413] -> w24
    tunnel: [w401] -> w16
    tunnel: w8 -> [w399]
    stop <- "Stop 9" stop-if-true
    w384 = 1 items=["one channel for each line", "one channel for all lines"] ("line grouping")
    w392 = 1 items=["one channel for each line", "one channel for all lines"] ("line grouping")
    w404 = 1 items=["one channel for each line", "one channel for all lines"] ("line grouping")
    w413 = 0.05 ("Sampling Time dt (s)")
    w421 = 1 items=["one channel for each line", "one channel for all lines"] ("line grouping")
    w429 = 0.5 ("x")
    w456 = T7 {"static gain"=2.5, "lag (s)"=2.5, "deadtime (s)"=0.01, "load"=0.0, "deadband"=0.0, "sensor noise"=0.0, "initial PV"=30.0, "plant noise"=0.0}  # Process parameters
    w458 = FALSE  # Integrator ?
    # "Inlet 11"
    # "Exhaust 3"
    # "C."
    # "Inlet 11"
    # "Exhaust 4"
    # "B."
    # "A."
    # "A.Output to PWM Logic \nB. Simulated Plant\nC. Draw Chart"
    # "Main PID Loop Control"
    n155 = Dequeue Element(queue=w399) -> (element=w400:dbl)  [unwired: 2 in, 3 out]
    n156 = Multiply(x=w413, y=1000.0) -> (x*y=w455:dbl)
    n157 = Not(x="Autotune 9") -> (.not. x?=w459:bool)
    n158 = feedback #4() -> (w464:bool)  [unwired: 1 in]
    n159 = feedback-in #4("Autotune 9") -> ()
    n160 = Wait Until Next ms Multiple(millisecond multiple=w455) -> ()  [unwired: 1 out]
    n161 = Exclusive Or(1:w464, 2:"Autotune 9") -> (0:w463:bool)
    n162 = feedback #5() -> (w461:dbl)  [unwired: 1 in]
    n163 = Multiply(x=w400, y=-1000.0) -> (x*y=w445:dbl)
    n164 = call <vilib>:"Median PtByPt.vi"("sample length"="Median sample length 18", "x"=w445) -> ("median"=w444:dbl)  [unwired: 2 in, 1 out]
    n165 = Square(x=w444) -> (x^2=w452:dbl)
    n166 = Multiply(x=w444, y=0.1121) -> (x*y=w448:dbl)
    n167 = Multiply(x=w452, y=0.0243) -> (x*y=w449:dbl)
    n168 = Add(x=w448, y=w449) -> (x+y=w447:dbl)
    n169 = Add(x=-235.77, y=w447) -> (x+y=w411:dbl)
    n170 = case shown="True" "Autotune 9" {
      tunnel: w413 -> [w479 _]
      tunnel: [w468 w484] -> w418
      tunnel: w462 -> [_ w483]
      tunnel: "PID Gains 9" -> [w478 _]
      tunnel: "Reinitialize 9" -> [w475 _]
      tunnel: w463 -> [w477 w482]
      tunnel: w461 -> [_ w486]
      tunnel: w411 -> [w471 _]
      tunnel: "Set Point 3,4" -> [w470 _]
      frame False {
        # "This code is to have 'bumpless' transfer from autotuning"
        n171 = Not(x=w477) -> (.not. x?=w474:bool)
        n172 = And(x="Automatic 9", y=w474) -> (x .and. y?=w476:bool)
        n173 = call-poly <vilib>:"PID Advanced.vi"("setpoint"=w470, "auto? (T)"=w476, "manual control"="MV: 9", "process variable"=w471, "alpha"=10.0, "PID gains"=w478, "dt (s)"=w479, "reinitialize? (F)"=w475) -> ("output"=w468:dbl)  [unwired: 6 in, 1 out]
      }
      frame True {
        w489 = 10000 ("sample length")
        # "Buffering data for parameters estimation"
        n174 = call <vilib>:"Data Queue PtByPt.vi"("initial queue element"=w483, "initialize"=w482, "sample length"=w489, "input data point"=w483) -> ("Current Queue"=→"Control Output 9":dbl[])  [unwired: 3 in, 4 out]
        n175 = Select(t=0.0, s=w482, f="Excitation 9") -> (s? t:f=w487:dbl)
        n176 = Add(x=w486, y=w487) -> (x+y=w484:dbl)
        n177 = call <vilib>:"Data Queue PtByPt.vi"("initial queue element"=w484, "initialize"=w482, "sample length"=w489, "input data point"=w484) -> ("Current Queue"=→"Measurement 9":dbl[])  [unwired: 3 in, 4 out]
      }
    }
    n178 = feedback-in #5(w418, w459) -> ()
    n179 = Greater?(x=w411, y="M-3,4") -> (0:w401:bool)
    n180 = Add(x=w441, y=w429) -> (x+y=w430:dbl)
    n181 = Subtract(x=w441, y=w429) -> (x-y=w428:dbl)
    n182 = Equal?(x=w439, y=w418) -> (x = y?=w436:bool)
    n183 = Greater?(x=w418, y=w439) -> (0:w435:bool)
    n184 = Select(t=w440, s=w436, f=w435) -> (s? t:f=w416:bool)
    "PWM Output 9" <- w416
    n185 = call "Plant System.vi"("Integrator ?"=w458, "Plant Input"=w418, "dt (s)"=w413, "process parameters"=w456) -> ("Plant Output"=w457:dbl)  [unwired: 11 in]
    n186 = Increment(x="Set Point 3,4") -> (x+1=w434:dbl)
    n187 = Decrement(x="Set Point 3,4") -> (x-1=w433:dbl)
    n188 = Select(t=w430, s=w416, f=w428) -> (s? t:f=w443:dbl)
    n189 = Select(t=w434, s=w416, f=w433) -> (s? t:f=w432:dbl)
    n190 = Not(x=w416) -> (.not. x?=w415:bool)
    n191 = call-poly <vilib>:"DAQmx Create Virtual Channel.vi"("lines"=tag "cDAQ1Mod8/port0/line5", "line grouping"=w421) -> ("task out"=w423:refnum<k21>, "error out"=w422:errorcluster)  [unwired: 12 in]
    n192 = call-poly <vilib>:"DAQmx Create Virtual Channel.vi"("lines"=tag "cDAQ1Mod7/port0/line4", "line grouping"=w404) -> ("task out"=w406:refnum<k21>, "error out"=w405:errorcluster)  [unwired: 12 in]
    n193 = Build Array(w411, "Set Point 3,4", w432) -> (w431:dbl[])
    n194 = Initialize Array("INLET 3,4 ON/OFF 2", 1 ("dimension size")) -> (w380:bool[])
    n195 = Initialize Array(w415, 1 ("dimension size")) -> (w382:bool[])
    n196 = local write "MV: 9"(w418) -> ()
    n197 = Add(x=w438, y=w441) -> (x+y=w442:dbl)
    n198 = Build Array(w431) -> (→"Real time Data 3,4":dbl[][])
    n199 = call-poly <vilib>:"DAQmx Write.vi"("task/channels in"=w423, "auto start"=TRUE, "data"=w382, "error in"=w422) -> ("task out"=w425:refnum<k21>, "error out"=w426:errorcluster)  [unwired: 9 in, 1 out]
    n200 = call-poly <vilib>:"DAQmx Write.vi"("task/channels in"=w406, "auto start"=TRUE, "data"=w380, "error in"=w405) -> ("task out"=w408:refnum<k21>, "error out"=w409:errorcluster)  [unwired: 9 in, 1 out]
    n201 = call <vilib>:"DAQmx Clear Task.vi"("task in"=w425, "error in"=w426) -> ("error out"=w420:errorcluster)  [unwired: 13 in]
    n202 = call <vilib>:"DAQmx Clear Task.vi"("task in"=w408, "error in"=w409) -> ("error out"=w403:errorcluster)  [unwired: 13 in]
    n203 = call <vilib>:"Simple Error Handler.vi"("error in (no error)"=w420) -> ()  [unwired: 4 in, 5 out]
    n204 = call <vilib>:"Simple Error Handler.vi"("error in (no error)"=w403) -> ()  [unwired: 4 in, 5 out]
    n205 = call-poly <vilib>:"DAQmx Create Virtual Channel.vi"("lines"=tag "cDAQ1Mod8/port0/line7", "line grouping"=w392) -> ("task out"=w394:refnum<k21>, "error out"=w393:errorcluster)  [unwired: 12 in]
    n206 = call-poly <vilib>:"DAQmx Create Virtual Channel.vi"("lines"=tag "cDAQ1Mod7/port0/line6", "line grouping"=w384) -> ("task out"=w386:refnum<k21>, "error out"=w385:errorcluster)  [unwired: 12 in]
    n207 = call-poly <vilib>:"DAQmx Write.vi"("task/channels in"=w394, "auto start"=TRUE, "data"=w382, "error in"=w393) -> ("task out"=w396:refnum<k21>, "error out"=w397:errorcluster)  [unwired: 9 in, 1 out]
    n208 = call-poly <vilib>:"DAQmx Write.vi"("task/channels in"=w386, "auto start"=TRUE, "data"=w380, "error in"=w385) -> ("task out"=w388:refnum<k21>, "error out"=w389:errorcluster)  [unwired: 9 in, 1 out]
    n209 = call <vilib>:"DAQmx Clear Task.vi"("task in"=w396, "error in"=w397) -> ("error out"=w391:errorcluster)  [unwired: 13 in]
    n210 = call <vilib>:"DAQmx Clear Task.vi"("task in"=w388, "error in"=w389) -> ("error out"=w383:errorcluster)  [unwired: 13 in]
    n211 = call <vilib>:"Simple Error Handler.vi"("error in (no error)"=w391) -> ()  [unwired: 4 in, 5 out]
    n212 = call <vilib>:"Simple Error Handler.vi"("error in (no error)"=w383) -> ()  [unwired: 4 in, 5 out]
  }
  n213 = control-ref of="stop"() -> (w67:refnum<vi>)
  n214 = control-ref of="XYZAER"() -> (w58:refnum<vi>)
  n215 = Obtain Queue(element data type=0.0) -> (queue out=w5:refnum<queue>)  [unwired: 4 in, 2 out]
  n216 = while {
    shift-left: 0.0 ("Plant Output") -> [w556]
    shift-right: [w551] -> _
    tunnel: w34 -> [_]
    shift-right: [w537] -> _
    shift-left: 0.01 -> [w535]
    shift-right: [w509] -> _
    shift-left: TRUE -> [w534]
    shift-right: [w511] -> _
    shift-left: w31 -> [w533]
    shift-right: [w536] -> _
    shift-left: w31 -> [w532]
    tunnel: [w506] -> w30
    tunnel: [w492] -> w15
    tunnel: w5 -> [w490]
    stop <- "Stop 8" stop-if-true
    w497 = 1 items=["one channel for each line", "one channel for all lines"] ("line grouping")
    w506 = 0.05 ("Sampling Time dt (s)")
    w515 = 1 items=["one channel for each line", "one channel for all lines"] ("line grouping")
    w523 = 0.5 ("x")
    w550 = T7 {"static gain"=2.5, "lag (s)"=2.5, "deadtime (s)"=0.01, "load"=0.0, "deadband"=0.0, "sensor noise"=0.0, "initial PV"=30.0, "plant noise"=0.0}  # Process parameters
    w552 = FALSE  # Integrator ?
    # "C."
    # "Inlet 11"
    # "Exhaust 2"
    # "B."
    # "A."
    # "A.Output to PWM Logic \nB. Simulated Plant\nC. Draw Chart"
    # "Main PID Loop Control"
    n217 = Dequeue Element(queue=w490) -> (element=w491:dbl)  [unwired: 2 in, 3 out]
    n218 = Multiply(x=w506, y=1000.0) -> (x*y=w549:dbl)
    n219 = Not(x="Autotune 8") -> (.not. x?=w553:bool)
    n220 = feedback #6() -> (w558:bool)  [unwired: 1 in]
    n221 = feedback-in #6("Autotune 8") -> ()
    n222 = Wait Until Next ms Multiple(millisecond multiple=w549) -> ()  [unwired: 1 out]
    n223 = Exclusive Or(1:w558, 2:"Autotune 8") -> (0:w557:bool)
    n224 = feedback #7() -> (w555:dbl)  [unwired: 1 in]
    n225 = Multiply(x=w491, y=-1000.0) -> (x*y=w539:dbl)
    n226 = call <vilib>:"Median PtByPt.vi"("sample length"="Median sample length 17", "x"=w539) -> ("median"=w538:dbl)  [unwired: 2 in, 1 out]
    n227 = Square(x=w538) -> (x^2=w546:dbl)
    n228 = Multiply(x=w538, y=-7.5945) -> (x*y=w542:dbl)
    n229 = Multiply(x=w546, y=0.0612) -> (x*y=w543:dbl)
    n230 = Add(x=w542, y=w543) -> (x+y=w541:dbl)
    n231 = Add(x=143.72, y=w541) -> (x+y=w504:dbl)
    n232 = case shown="False" "Autotune 8" {
      tunnel: w506 -> [w573 _]
      tunnel: [w562 w578] -> w511
      tunnel: w556 -> [_ w577]
      tunnel: "PID Gains 8" -> [w572 _]
      tunnel: "Reinitialize 8" -> [w569 _]
      tunnel: w557 -> [w571 w576]
      tunnel: w555 -> [_ w580]
      tunnel: w504 -> [w565 _]
      tunnel: "Set Point 2" -> [w564 _]
      frame False {
        # "This code is to have 'bumpless' transfer from autotuning"
        n233 = Not(x=w571) -> (.not. x?=w568:bool)
        n234 = And(x="Automatic 8", y=w568) -> (x .and. y?=w570:bool)
        n235 = call-poly <vilib>:"PID Advanced.vi"("setpoint"=w564, "auto? (T)"=w570, "manual control"="MV: 8", "process variable"=w565, "alpha"=10.0, "PID gains"=w572, "dt (s)"=w573, "reinitialize? (F)"=w569) -> ("output"=w562:dbl)  [unwired: 6 in, 1 out]
      }
      frame True {
        w583 = 10000 ("sample length")
        # "Buffering data for parameters estimation"
        n236 = call <vilib>:"Data Queue PtByPt.vi"("initial queue element"=w577, "initialize"=w576, "sample length"=w583, "input data point"=w577) -> ("Current Queue"=→"Control Output 8":dbl[])  [unwired: 3 in, 4 out]
        n237 = Select(t=0.0, s=w576, f="Excitation 8") -> (s? t:f=w581:dbl)
        n238 = Add(x=w580, y=w581) -> (x+y=w578:dbl)
        n239 = call <vilib>:"Data Queue PtByPt.vi"("initial queue element"=w578, "initialize"=w576, "sample length"=w583, "input data point"=w578) -> ("Current Queue"=→"Measurement 8":dbl[])  [unwired: 3 in, 4 out]
      }
    }
    n240 = feedback-in #7(w511, w553) -> ()
    n241 = Greater?(x=w504, y="M-2") -> (0:w492:bool)
    n242 = Add(x=w535, y=w523) -> (x+y=w524:dbl)
    n243 = Subtract(x=w535, y=w523) -> (x-y=w522:dbl)
    n244 = Equal?(x=w533, y=w511) -> (x = y?=w530:bool)
    n245 = Greater?(x=w511, y=w533) -> (0:w529:bool)
    n246 = Select(t=w534, s=w530, f=w529) -> (s? t:f=w509:bool)
    "PWM Output 8" <- w509
    n247 = call "Plant System.vi"("Integrator ?"=w552, "Plant Input"=w511, "dt (s)"=w506, "process parameters"=w550) -> ("Plant Output"=w551:dbl)  [unwired: 11 in]
    n248 = Increment(x="Set Point 2") -> (x+1=w528:dbl)
    n249 = Decrement(x="Set Point 2") -> (x-1=w527:dbl)
    n250 = Select(t=w524, s=w509, f=w522) -> (s? t:f=w537:dbl)
    n251 = Select(t=w528, s=w509, f=w527) -> (s? t:f=w526:dbl)
    n252 = Not(x=w509) -> (.not. x?=w508:bool)
    n253 = call-poly <vilib>:"DAQmx Create Virtual Channel.vi"("lines"=tag "cDAQ1Mod1/port0/line6", "line grouping"=w515) -> ("task out"=w517:refnum<k21>, "error out"=w516:errorcluster)  [unwired: 12 in]
    n254 = call-poly <vilib>:"DAQmx Create Virtual Channel.vi"("lines"=tag "cDAQ1Mod2/port0/line6", "line grouping"=w497) -> ("task out"=w499:refnum<k21>, "error out"=w498:errorcluster)  [unwired: 12 in]
    n255 = Build Array(w504, "Set Point 2", w526) -> (w525:dbl[])
    n256 = Initialize Array("INLET 2 ON/OFF 2", 1 ("dimension size")) -> (w494:bool[])
    n257 = Initialize Array(w508, 1 ("dimension size")) -> (w512:bool[])
    n258 = local write "MV: 8"(w511) -> ()
    n259 = Add(x=w532, y=w535) -> (x+y=w536:dbl)
    n260 = Build Array(w525) -> (→"Real time Data 2":dbl[][])
    n261 = call-poly <vilib>:"DAQmx Write.vi"("task/channels in"=w517, "auto start"=TRUE, "data"=w512, "error in"=w516) -> ("task out"=w519:refnum<k21>, "error out"=w520:errorcluster)  [unwired: 9 in, 1 out]
    n262 = call-poly <vilib>:"DAQmx Write.vi"("task/channels in"=w499, "auto start"=TRUE, "data"=w494, "error in"=w498) -> ("task out"=w501:refnum<k21>, "error out"=w502:errorcluster)  [unwired: 9 in, 1 out]
    n263 = call <vilib>:"DAQmx Clear Task.vi"("task in"=w519, "error in"=w520) -> ("error out"=w514:errorcluster)  [unwired: 13 in]
    n264 = call <vilib>:"DAQmx Clear Task.vi"("task in"=w501, "error in"=w502) -> ("error out"=w496:errorcluster)  [unwired: 13 in]
    n265 = call <vilib>:"Simple Error Handler.vi"("error in (no error)"=w514) -> ()  [unwired: 4 in, 5 out]
    n266 = call <vilib>:"Simple Error Handler.vi"("error in (no error)"=w496) -> ()  [unwired: 4 in, 5 out]
  }
  n267 = Obtain Queue(element data type=0.0) -> (queue out=w4:refnum<queue>)  [unwired: 4 in, 2 out]
  n268 = while {
    shift-left: 0.0 ("Plant Output") -> [w650]
    shift-right: [w645] -> _
    tunnel: w40 -> [_]
    shift-right: [w631] -> _
    shift-left: 0.01 -> [w629]
    shift-right: [w603] -> _
    shift-left: TRUE -> [w628]
    shift-right: [w605] -> _
    shift-left: w37 -> [w627]
    shift-right: [w630] -> _
    shift-left: w37 -> [w626]
    tunnel: [w600] -> w36
    tunnel: [w586] -> w14
    tunnel: w4 -> [w584]
    stop <- "Stop 7" stop-if-true
    w591 = 1 items=["one channel for each line", "one channel for all lines"] ("line grouping")
    w600 = 0.05 ("Sampling Time dt (s)")
    w609 = 1 items=["one channel for each line", "one channel for all lines"] ("line grouping")
    w617 = 0.5 ("x")
    w644 = T7 {"static gain"=2.5, "lag (s)"=2.5, "deadtime (s)"=0.01, "load"=0.0, "deadband"=0.0, "sensor noise"=0.0, "initial PV"=30.0, "plant noise"=0.0}  # Process parameters
    w646 = FALSE  # Integrator ?
    # "C."
    # "Inlet 11"
    # "Exhaust 7"
    # "B."
    # "A."
    # "A.Output to PWM Logic \nB. Simulated Plant\nC. Draw Chart"
    # "Main PID Loop Control"
    n269 = Dequeue Element(queue=w584) -> (element=w585:dbl)  [unwired: 2 in, 3 out]
    n270 = Multiply(x=w600, y=1000.0) -> (x*y=w643:dbl)
    n271 = Not(x="Autotune 7") -> (.not. x?=w647:bool)
    n272 = feedback #8() -> (w652:bool)  [unwired: 1 in]
    n273 = feedback-in #8("Autotune 7") -> ()
    n274 = Wait Until Next ms Multiple(millisecond multiple=w643) -> ()  [unwired: 1 out]
    n275 = Exclusive Or(1:w652, 2:"Autotune 7") -> (0:w651:bool)
    n276 = feedback #9() -> (w649:dbl)  [unwired: 1 in]
    n277 = Multiply(x=w585, y=-1000.0) -> (x*y=w633:dbl)
    n278 = call <vilib>:"Median PtByPt.vi"("sample length"="Median sample length 16", "x"=w633) -> ("median"=w632:dbl)  [unwired: 2 in, 1 out]
    n279 = Square(x=w632) -> (x^2=w640:dbl)
    n280 = Multiply(x=w632, y=-0.6707) -> (x*y=w636:dbl)
    n281 = Multiply(x=w640, y=0.0015) -> (x*y=w637:dbl)
    n282 = Add(x=w636, y=w637) -> (x+y=w635:dbl)
    n283 = Add(x=-0.8771, y=w635) -> (x+y=w598:dbl)
    n284 = case shown="False" "Autotune 7" {
      tunnel: w600 -> [w667 _]
      tunnel: [w656 w672] -> w605
      tunnel: w650 -> [_ w671]
      tunnel: "PID Gains 7" -> [w666 _]
      tunnel: "Reinitialize 7" -> [w663 _]
      tunnel: w651 -> [w665 w670]
      tunnel: w649 -> [_ w674]
      tunnel: w598 -> [w659 _]
      tunnel: "Set Point 7" -> [w658 _]
      frame False {
        # "This code is to have 'bumpless' transfer from autotuning"
        n285 = Not(x=w665) -> (.not. x?=w662:bool)
        n286 = And(x="Automatic 7", y=w662) -> (x .and. y?=w664:bool)
        n287 = call-poly <vilib>:"PID Advanced.vi"("setpoint"=w658, "auto? (T)"=w664, "manual control"="MV: 7", "process variable"=w659, "alpha"=10.0, "PID gains"=w666, "dt (s)"=w667, "reinitialize? (F)"=w663) -> ("output"=w656:dbl)  [unwired: 6 in, 1 out]
      }
      frame True {
        w677 = 10000 ("sample length")
        # "Buffering data for parameters estimation"
        n288 = call <vilib>:"Data Queue PtByPt.vi"("initial queue element"=w671, "initialize"=w670, "sample length"=w677, "input data point"=w671) -> ("Current Queue"=→"Control Output 7":dbl[])  [unwired: 3 in, 4 out]
        n289 = Select(t=0.0, s=w670, f="Excitation 7") -> (s? t:f=w675:dbl)
        n290 = Add(x=w674, y=w675) -> (x+y=w672:dbl)
        n291 = call <vilib>:"Data Queue PtByPt.vi"("initial queue element"=w672, "initialize"=w670, "sample length"=w677, "input data point"=w672) -> ("Current Queue"=→"Measurement 7":dbl[])  [unwired: 3 in, 4 out]
      }
    }
    n292 = feedback-in #9(w605, w647) -> ()
    n293 = Greater?(x=w598, y="M-7") -> (0:w586:bool)
    n294 = Add(x=w629, y=w617) -> (x+y=w618:dbl)
    n295 = Subtract(x=w629, y=w617) -> (x-y=w616:dbl)
    n296 = Equal?(x=w627, y=w605) -> (x = y?=w624:bool)
    n297 = Greater?(x=w605, y=w627) -> (0:w623:bool)
    n298 = Select(t=w628, s=w624, f=w623) -> (s? t:f=w603:bool)
    "PWM Output 7" <- w603
    n299 = call "Plant System.vi"("Integrator ?"=w646, "Plant Input"=w605, "dt (s)"=w600, "process parameters"=w644) -> ("Plant Output"=w645:dbl)  [unwired: 11 in]
    n300 = Increment(x="Set Point 7") -> (x+1=w622:dbl)
    n301 = Decrement(x="Set Point 7") -> (x-1=w621:dbl)
    n302 = Select(t=w618, s=w603, f=w616) -> (s? t:f=w631:dbl)
    n303 = Select(t=w622, s=w603, f=w621) -> (s? t:f=w620:dbl)
    n304 = Not(x=w603) -> (.not. x?=w602:bool)
    n305 = call-poly <vilib>:"DAQmx Create Virtual Channel.vi"("lines"=tag "cDAQ1Mod8/port0/line4", "line grouping"=w609) -> ("task out"=w611:refnum<k21>, "error out"=w610:errorcluster)  [unwired: 12 in]
    n306 = call-poly <vilib>:"DAQmx Create Virtual Channel.vi"("lines"=tag "cDAQ1Mod7/port0/line3", "line grouping"=w591) -> ("task out"=w593:refnum<k21>, "error out"=w592:errorcluster)  [unwired: 12 in]
    n307 = Build Array(w598, "Set Point 7", w620) -> (w619:dbl[])
    n308 = Initialize Array("INLET 7 ON/OFF 2", 1 ("dimension size")) -> (w588:bool[])
    n309 = Initialize Array(w602, 1 ("dimension size")) -> (w606:bool[])
    n310 = local write "MV: 7"(w605) -> ()
    n311 = Add(x=w626, y=w629) -> (x+y=w630:dbl)
    n312 = Build Array(w619) -> (→"Real time Data 7":dbl[][])
    n313 = call-poly <vilib>:"DAQmx Write.vi"("task/channels in"=w611, "auto start"=TRUE, "data"=w606, "error in"=w610) -> ("task out"=w613:refnum<k21>, "error out"=w614:errorcluster)  [unwired: 9 in, 1 out]
    n314 = call-poly <vilib>:"DAQmx Write.vi"("task/channels in"=w593, "auto start"=TRUE, "data"=w588, "error in"=w592) -> ("task out"=w595:refnum<k21>, "error out"=w596:errorcluster)  [unwired: 9 in, 1 out]
    n315 = call <vilib>:"DAQmx Clear Task.vi"("task in"=w613, "error in"=w614) -> ("error out"=w608:errorcluster)  [unwired: 13 in]
    n316 = call <vilib>:"DAQmx Clear Task.vi"("task in"=w595, "error in"=w596) -> ("error out"=w590:errorcluster)  [unwired: 13 in]
    n317 = call <vilib>:"Simple Error Handler.vi"("error in (no error)"=w608) -> ()  [unwired: 4 in, 5 out]
    n318 = call <vilib>:"Simple Error Handler.vi"("error in (no error)"=w590) -> ()  [unwired: 4 in, 5 out]
  }
  n319 = Obtain Queue(element data type=0.0) -> (queue out=w10:refnum<queue>)  [unwired: 4 in, 2 out]
  n320 = while {
    shift-left: 0.0 ("Plant Output") -> [w777]
    shift-right: [w772] -> _
    tunnel: w88 -> [_]
    shift-right: [w758] -> _
    shift-left: 0.01 -> [w756]
    shift-right: [w731] -> _
    shift-left: TRUE -> [w755]
    shift-right: [w733] -> _
    shift-left: w85 -> [w754]
    shift-right: [w757] -> _
    shift-left: w85 -> [w753]
    tunnel: [w728] -> w84
    tunnel: [w725] -> w1
    tunnel: w12 -> [w702]
    tunnel: w10 -> [w701]
    tunnel: w8 -> [w700]
    tunnel: w5 -> [w697]
    tunnel: w4 -> [w696]
    stop <- "Stop" stop-if-true
    w681 = 1 items=["one channel for each line", "one channel for all lines"] ("line grouping")
    w689 = 1 items=["one channel for each line", "one channel for all lines"] ("line grouping")
    w718 = 1 items=["one channel for each line", "one channel for all lines"] ("line grouping")
    w728 = 0.05 ("Sampling Time dt (s)")
    w736 = 1 items=["one channel for each line", "one channel for all lines"] ("line grouping")
    w744 = 0.5 ("x")
    w771 = T7 {"static gain"=2.5, "lag (s)"=2.5, "deadtime (s)"=0.01, "load"=0.0, "deadband"=0.0, "sensor noise"=0.0, "initial PV"=30.0, "plant noise"=0.0}  # Process parameters
    w773 = FALSE  # Integrator ?
    # "Inlet 11"
    # "Exhaust 12"
    # "C."
    # "Inlet 11"
    # "Exhaust 11"
    # "B."
    # "A."
    # "A.Output to PWM Logic \nB. Simulated Plant\nC. Draw Chart"
    # "Main PID Loop Control"
    n321 = call-poly <vilib>:"DAQmx Read.vi"("task/channels in"=refnum<k21> "1_4_2_7_6_5") -> ("data"=w708:dbl[])  [unwired: 12 in, 2 out]
    n322 = Index Array(array=w708, index=0) -> (element=w703:dbl)
    n323 = Index Array(array=w708, index=1) -> (element=w704:dbl)
    n324 = Index Array(array=w708, index=2) -> (element=w699:dbl)
    n325 = Index Array(array=w708, index=5) -> (element=w706:dbl)
    n326 = Index Array(array=w708, index=4) -> (element=w705:dbl)
    n327 = Index Array(array=w708, index=3) -> (element=w698:dbl)
    n328 = Enqueue Element(queue=w701, element=w703) -> ()  [unwired: 2 in, 3 out]
    n329 = Enqueue Element(queue=w697, element=w699) -> ()  [unwired: 2 in, 3 out]
    n330 = Multiply(x=w728, y=1000.0) -> (x*y=w770:dbl)
    n331 = Enqueue Element(queue=w700, element=w704) -> ()  [unwired: 2 in, 3 out]
    n332 = Not(x="Autotune") -> (.not. x?=w774:bool)
    n333 = feedback #10() -> (w779:bool)  [unwired: 1 in]
    n334 = feedback-in #10("Autotune") -> ()
    n335 = Enqueue Element(queue=w696, element=w698) -> ()  [unwired: 2 in, 3 out]
    n336 = Wait Until Next ms Multiple(millisecond multiple=w770) -> ()  [unwired: 1 out]
    n337 = Exclusive Or(1:w779, 2:"Autotune") -> (0:w778:bool)
    n338 = feedback #11() -> (w776:dbl)  [unwired: 1 in]
    n339 = Enqueue Element(queue=w702, element=w705) -> ()  [unwired: 2 in, 3 out]
    n340 = Multiply(x=w706, y=-1000.0) -> (x*y=w760:dbl)
    n341 = call <vilib>:"Median PtByPt.vi"("sample length"="Median sample length", "x"=w760) -> ("median"=w759:dbl)  [unwired: 2 in, 1 out]
    n342 = Square(x=w759) -> (x^2=w767:dbl)
    n343 = Multiply(x=w759, y=-39.646) -> (x*y=w763:dbl)
    n344 = Multiply(x=w767, y=0.2324) -> (x*y=w764:dbl)
    n345 = Add(x=w763, y=w764) -> (x+y=w762:dbl)
    n346 = Add(x=1678.0, y=w762) -> (x+y=w726:dbl)
    n347 = case shown="False" "Autotune" {
      tunnel: w728 -> [w794 _]
      tunnel: [w783 w799] -> w733
      tunnel: w777 -> [_ w798]
      tunnel: "PID Gains" -> [w793 _]
      tunnel: "Reinitialize" -> [w790 _]
      tunnel: w778 -> [w792 w797]
      tunnel: w776 -> [_ w801]
      tunnel: w726 -> [w786 _]
      tunnel: "Set Point 11,12" -> [w785 _]
      frame False {
        # "This code is to have 'bumpless' transfer from autotuning"
        n348 = Not(x=w792) -> (.not. x?=w789:bool)
        n349 = And(x="Automatic", y=w789) -> (x .and. y?=w791:bool)
        n350 = call-poly <vilib>:"PID Advanced.vi"("setpoint"=w785, "auto? (T)"=w791, "manual control"="MV:", "process variable"=w786, "alpha"=10.0, "PID gains"=w793, "dt (s)"=w794, "reinitialize? (F)"=w790) -> ("output"=w783:dbl)  [unwired: 6 in, 1 out]
      }
      frame True {
        w804 = 10000 ("sample length")
        # "Buffering data for parameters estimation"
        n351 = call <vilib>:"Data Queue PtByPt.vi"("initial queue element"=w798, "initialize"=w797, "sample length"=w804, "input data point"=w798) -> ("Current Queue"=→"Control Output":dbl[])  [unwired: 3 in, 4 out]
        n352 = Select(t=0.0, s=w797, f="Excitation") -> (s? t:f=w802:dbl)
        n353 = Add(x=w801, y=w802) -> (x+y=w799:dbl)
        n354 = call <vilib>:"Data Queue PtByPt.vi"("initial queue element"=w799, "initialize"=w797, "sample length"=w804, "input data point"=w799) -> ("Current Queue"=→"Measurement":dbl[])  [unwired: 3 in, 4 out]
      }
    }
    n355 = feedback-in #11(w733, w774) -> ()
    n356 = Greater?(x=w726, y="M-11,12") -> (0:w725:bool)
    n357 = Add(x=w756, y=w744) -> (x+y=w745:dbl)
    n358 = Subtract(x=w756, y=w744) -> (x-y=w743:dbl)
    n359 = Equal?(x=w754, y=w733) -> (x = y?=w751:bool)
    n360 = Greater?(x=w733, y=w754) -> (0:w750:bool)
    n361 = Select(t=w755, s=w751, f=w750) -> (s? t:f=w731:bool)
    "PWM Output" <- w731
    n362 = call "Plant System.vi"("Integrator ?"=w773, "Plant Input"=w733, "dt (s)"=w728, "process parameters"=w771) -> ("Plant Output"=w772:dbl)  [unwired: 11 in]
    n363 = Increment(x="Set Point 11,12") -> (x+1=w749:dbl)
    n364 = Decrement(x="Set Point 11,12") -> (x-1=w748:dbl)
    n365 = Select(t=w745, s=w731, f=w743) -> (s? t:f=w758:dbl)
    n366 = Select(t=w749, s=w731, f=w748) -> (s? t:f=w747:dbl)
    n367 = Not(x=w731) -> (.not. x?=w730:bool)
    n368 = call-poly <vilib>:"DAQmx Create Virtual Channel.vi"("lines"=tag "cDAQ1Mod1/port0/line2", "line grouping"=w736) -> ("task out"=w738:refnum<k21>, "error out"=w737:errorcluster)  [unwired: 12 in]
    n369 = call-poly <vilib>:"DAQmx Create Virtual Channel.vi"("lines"=tag "cDAQ1Mod2/port0/line2", "line grouping"=w718) -> ("task out"=w720:refnum<k21>, "error out"=w719:errorcluster)  [unwired: 12 in]
    n370 = Build Array(w726, "Set Point 11,12", w747) -> (w746:dbl[])
    n371 = Initialize Array("INLET", 1 ("dimension size")) -> (w678:bool[])
    n372 = Initialize Array(w730, 1 ("dimension size")) -> (w679:bool[])
    n373 = call-poly <vilib>:"DAQmx Create Virtual Channel.vi"("lines"=tag "cDAQ1Mod8/port0/line2", "line grouping"=w689) -> ("task out"=w691:refnum<k21>, "error out"=w690:errorcluster)  [unwired: 12 in]
    n374 = call-poly <vilib>:"DAQmx Create Virtual Channel.vi"("lines"=tag "cDAQ1Mod7/port0/line1", "line grouping"=w681) -> ("task out"=w683:refnum<k21>, "error out"=w682:errorcluster)  [unwired: 12 in]
    n375 = local write "MV:"(w733) -> ()
    n376 = Add(x=w753, y=w756) -> (x+y=w757:dbl)
    n377 = Build Array(w746) -> (→"Real time Data -11,12":dbl[][])
    n378 = call-poly <vilib>:"DAQmx Write.vi"("task/channels in"=w738, "auto start"=TRUE, "data"=w679, "error in"=w737) -> ("task out"=w740:refnum<k21>, "error out"=w741:errorcluster)  [unwired: 9 in, 1 out]
    n379 = call-poly <vilib>:"DAQmx Write.vi"("task/channels in"=w720, "auto start"=TRUE, "data"=w678, "error in"=w719) -> ("task out"=w722:refnum<k21>, "error out"=w723:errorcluster)  [unwired: 9 in, 1 out]
    n380 = call-poly <vilib>:"DAQmx Write.vi"("task/channels in"=w691, "auto start"=TRUE, "data"=w679, "error in"=w690) -> ("task out"=w693:refnum<k21>, "error out"=w694:errorcluster)  [unwired: 9 in, 1 out]
    n381 = call-poly <vilib>:"DAQmx Write.vi"("task/channels in"=w683, "auto start"=TRUE, "data"=w678, "error in"=w682) -> ("task out"=w685:refnum<k21>, "error out"=w686:errorcluster)  [unwired: 9 in, 1 out]
    n382 = call <vilib>:"DAQmx Clear Task.vi"("task in"=w740, "error in"=w741) -> ("error out"=w735:errorcluster)  [unwired: 13 in]
    n383 = call <vilib>:"DAQmx Clear Task.vi"("task in"=w722, "error in"=w723) -> ("error out"=w717:errorcluster)  [unwired: 13 in]
    n384 = call <vilib>:"DAQmx Clear Task.vi"("task in"=w693, "error in"=w694) -> ("error out"=w688:errorcluster)  [unwired: 13 in]
    n385 = call <vilib>:"DAQmx Clear Task.vi"("task in"=w685, "error in"=w686) -> ("error out"=w680:errorcluster)  [unwired: 13 in]
    n386 = call <vilib>:"Simple Error Handler.vi"("error in (no error)"=w735) -> ()  [unwired: 4 in, 5 out]
    n387 = call <vilib>:"Simple Error Handler.vi"("error in (no error)"=w717) -> ()  [unwired: 4 in, 5 out]
    n388 = call <vilib>:"Simple Error Handler.vi"("error in (no error)"=w688) -> ()  [unwired: 4 in, 5 out]
    n389 = call <vilib>:"Simple Error Handler.vi"("error in (no error)"=w680) -> ()  [unwired: 4 in, 5 out]
  }
  n390 = while {
    tunnel: w88 -> [_]
    tunnel: w84 -> [w808]
    stop <- w818 stop-if-true
    # "If dT and deadtime have similar values, the identification could evaluate deadtime as zero and this generates proportional gain equal to Inf. This code avoid gain changes in this situations."
    # "Autotuning Loop"
    n391 = local read "Control Output"() -> (w820:dbl[])
    n392 = local read "Measurement"() -> (w819:dbl[])
    n393 = case shown="\"Chien-Hrones-Reswick\"" "Control" {
      tunnel: w820 -> [w829 w837 w846 w855]
      tunnel: w819 -> [w828 w836 w845 w854]
      tunnel: [w827 w835 w844 w853] -> w807
      tunnel: [w826 w834 w843 w852] -> w806
      tunnel: w808 -> [w825 w833 w842 w851]
      tunnel: [w824 w832 w841 w850] -> w805
      tunnel: [w823 w831 w840 w849] -> w810
      tunnel: "Type of controller" -> [w822 w830 w839 w848]
      frame "Ziegler-Nichols", Default {
        n394 = call-poly <vilib>:"PID Autotuning Design.vi"("Ziegler-Nichols Speed"="Ziegler-Nichols speed", "Type of Controller"=w822, "dt (s)"=w825, "Response signal"=w828, "Stimulus signal"=w829) -> ("PID gains"=w823:T3, "response operating point"=w826:dbl, "stimulus operating point"=w827:dbl, "Plant Parameters"=w824:T5)  [unwired: 3 in]
      }
      frame "Cohen-Coon" {
        n395 = call-poly <vilib>:"PID Autotuning Design.vi"("Type of Controller"=w830, "dt (s)"=w833, "Response signal"=w836, "Stimulus signal"=w837) -> ("PID gains"=w831:T3, "response offset"=w834:dbl, "stimulus offset"=w835:dbl, "Plant Parameters"=w832:T5)  [unwired: 4 in]
      }
      frame "Chien-Hrones-Reswick" {
        n396 = call-poly <vilib>:"PID Autotuning Design.vi"("Tuning specifications"="Tuning specifications", "Type of Controller"=w839, "dt (s)"=w842, "Response signal"=w845, "Stimulus signal"=w846) -> ("PID gains"=w840:T3, "response offset"=w843:dbl, "stimulus offset"=w844:dbl, "Plant Parameters"=w841:T5)  [unwired: 3 in]
      }
      frame "Internal Model Control" {
        n397 = call-poly <vilib>:"PID Autotuning Design.vi"("Desired Time Constant (tau_c)"="Multiplicative factor", "Type of Controller"=w848, "dt (s)"=w851, "Response signal"=w854, "Stimulus signal"=w855) -> ("PID gains"=w849:T3, "response offset"=w852:dbl, "stimulus offset"=w853:dbl, "Plant Parameters"=w850:T5)  [unwired: 3 in]
      }
    }
    "Stimulus operating point" <- w807
    "Response operating point" <- w806
    "Identified Plant Parameters" <- w805
    n398 = Unbundle(w810) -> ("proportional gain (Kc)"=w813:dbl)  [unwired: 2 out]
    n399 = Equal?(x=w813, y=inf) -> (x = y?=w812:bool)
    n400 = feedback #12() -> (w811:T3)  [unwired: 1 in]
    n401 = Select(t=w811, s=w812, f=w810) -> (s? t:f=w809:T3)
    "Tuned PID gains" <- w809
    n402 = feedback-in #12(w809) -> ()
    n403 = case shown="True" "Accept gain" {
      tunnel: w809 -> [_ w856]
      frame False {
      }
      frame True {
        n404 = local write "PID Gains"(w856) -> ()
      }
    }
    n405 = local read "Stop"() -> (w818:bool)
  }
  n406 = while {
    shift-left: 0.0 ("Plant Output") -> [w941]
    shift-right: [w936] -> _
    tunnel: w22 -> [_]
    shift-right: [w922] -> _
    shift-left: 0.01 -> [w920]
    shift-right: [w895] -> _
    shift-left: TRUE -> [w919]
    shift-right: [w897] -> _
    shift-left: w19 -> [w918]
    shift-right: [w921] -> _
    shift-left: w19 -> [w917]
    tunnel: [w892] -> w18
    tunnel: [w879] -> w3
    tunnel: w10 -> [w877]
    stop <- "Stop 12" stop-if-true
    w862 = 1 items=["one channel for each line", "one channel for all lines"] ("line grouping")
    w870 = 1 items=["one channel for each line", "one channel for all lines"] ("line grouping")
    w883 = 1 items=["one channel for each line", "one channel for all lines"] ("line grouping")
    w892 = 0.05 ("Sampling Time dt (s)")
    w900 = 1 items=["one channel for each line", "one channel for all lines"] ("line grouping")
    w908 = 0.5 ("x")
    w935 = T7 {"static gain"=2.5, "lag (s)"=2.5, "deadtime (s)"=0.01, "load"=0.0, "deadband"=0.0, "sensor noise"=0.0, "initial PV"=30.0, "plant noise"=0.0}  # Process parameters
    w937 = FALSE  # Integrator ?
    # "Inlet 11"
    # "Exhaust 5"
    # "C."
    # "Inlet 11"
    # "Exhaust 1"
    # "B."
    # "A."
    # "A.Output to PWM Logic \nB. Simulated Plant\nC. Draw Chart"
    # "Main PID Loop Control"
    n407 = Dequeue Element(queue=w877) -> (element=w878:dbl)  [unwired: 2 in, 3 out]
    n408 = Multiply(x=w892, y=1000.0) -> (x*y=w934:dbl)
    n409 = Not(x="Autotune 12") -> (.not. x?=w938:bool)
    n410 = feedback #13() -> (w943:bool)  [unwired: 1 in]
    n411 = feedback-in #13("Autotune 12") -> ()
    n412 = Wait Until Next ms Multiple(millisecond multiple=w934) -> ()  [unwired: 1 out]
    n413 = Exclusive Or(1:w943, 2:"Autotune 12") -> (0:w942:bool)
    n414 = feedback #14() -> (w940:dbl)  [unwired: 1 in]
    n415 = Multiply(x=w878, y=-1000.0) -> (x*y=w924:dbl)
    n416 = call <vilib>:"Median PtByPt.vi"("sample length"="Median sample length 21", "x"=w924) -> ("median"=w923:dbl)  [unwired: 2 in, 1 out]
    n417 = Square(x=w923) -> (x^2=w931:dbl)
    n418 = Multiply(x=w923, y=2.7367) -> (x*y=w927:dbl)
    n419 = Multiply(x=w931, y=0.0108) -> (x*y=w928:dbl)
    n420 = Add(x=w927, y=w928) -> (x+y=w926:dbl)
    n421 = Add(x=-331.61, y=w926) -> (x+y=w890:dbl)
    n422 = case shown="True" "Autotune 12" {
      tunnel: w892 -> [w958 _]
      tunnel: [w947 w963] -> w897
      tunnel: w941 -> [_ w962]
      tunnel: "PID Gains 12" -> [w957 _]
      tunnel: "Reinitialize 12" -> [w954 _]
      tunnel: w942 -> [w956 w961]
      tunnel: w940 -> [_ w965]
      tunnel: w890 -> [w950 _]
      tunnel: "Set Point 1,5" -> [w949 _]
      frame False {
        # "This code is to have 'bumpless' transfer from autotuning"
        n423 = Not(x=w956) -> (.not. x?=w953:bool)
        n424 = And(x="Automatic 12", y=w953) -> (x .and. y?=w955:bool)
        n425 = call-poly <vilib>:"PID Advanced.vi"("setpoint"=w949, "auto? (T)"=w955, "manual control"="MV: 12", "process variable"=w950, "alpha"=10.0, "PID gains"=w957, "dt (s)"=w958, "reinitialize? (F)"=w954) -> ("output"=w947:dbl)  [unwired: 6 in, 1 out]
      }
      frame True {
        w968 = 10000 ("sample length")
        # "Buffering data for parameters estimation"
        n426 = call <vilib>:"Data Queue PtByPt.vi"("initial queue element"=w962, "initialize"=w961, "sample length"=w968, "input data point"=w962) -> ("Current Queue"=→"Control Output 12":dbl[])  [unwired: 3 in, 4 out]
        n427 = Select(t=0.0, s=w961, f="Excitation 12") -> (s? t:f=w966:dbl)
        n428 = Add(x=w965, y=w966) -> (x+y=w963:dbl)
        n429 = call <vilib>:"Data Queue PtByPt.vi"("initial queue element"=w963, "initialize"=w961, "sample length"=w968, "input data point"=w963) -> ("Current Queue"=→"Measurement 12":dbl[])  [unwired: 3 in, 4 out]
      }
    }
    n430 = feedback-in #14(w897, w938) -> ()
    n431 = Greater?(x=w890, y="M-1,5") -> (0:w879:bool)
    n432 = Add(x=w920, y=w908) -> (x+y=w909:dbl)
    n433 = Subtract(x=w920, y=w908) -> (x-y=w907:dbl)
    n434 = Equal?(x=w918, y=w897) -> (x = y?=w915:bool)
    n435 = Greater?(x=w897, y=w918) -> (0:w914:bool)
    n436 = Select(t=w919, s=w915, f=w914) -> (s? t:f=w895:bool)
    "PWM Output 12" <- w895
    n437 = call "Plant System.vi"("Integrator ?"=w937, "Plant Input"=w897, "dt (s)"=w892, "process parameters"=w935) -> ("Plant Output"=w936:dbl)  [unwired: 11 in]
    n438 = Increment(x="Set Point 1,5") -> (x+1=w913:dbl)
    n439 = Decrement(x="Set Point 1,5") -> (x-1=w912:dbl)
    n440 = Select(t=w909, s=w895, f=w907) -> (s? t:f=w922:dbl)
    n441 = Select(t=w913, s=w895, f=w912) -> (s? t:f=w911:dbl)
    n442 = Not(x=w895) -> (.not. x?=w894:bool)
    n443 = call-poly <vilib>:"DAQmx Create Virtual Channel.vi"("lines"=tag "cDAQ1Mod1/port0/line7", "line grouping"=w900) -> ("task out"=w902:refnum<k21>, "error out"=w901:errorcluster)  [unwired: 12 in]
    n444 = call-poly <vilib>:"DAQmx Create Virtual Channel.vi"("lines"=tag "cDAQ1Mod2/port0/line7", "line grouping"=w883) -> ("task out"=w885:refnum<k21>, "error out"=w884:errorcluster)  [unwired: 12 in]
    n445 = Build Array(w890, "Set Point 1,5", w911) -> (w910:dbl[])
    n446 = Initialize Array("INLET 1,5 ON/OFF 3", 1 ("dimension size")) -> (w880:bool[])
    n447 = Initialize Array(w894, 1 ("dimension size")) -> (w857:bool[])
    n448 = local write "MV: 12"(w897) -> ()
    n449 = Add(x=w917, y=w920) -> (x+y=w921:dbl)
    n450 = Build Array(w910) -> (→"Real time Data 1,5":dbl[][])
    n451 = call-poly <vilib>:"DAQmx Write.vi"("task/channels in"=w902, "auto start"=TRUE, "data"=w857, "error in"=w901) -> ("task out"=w904:refnum<k21>, "error out"=w905:errorcluster)  [unwired: 9 in, 1 out]
    n452 = call-poly <vilib>:"DAQmx Write.vi"("task/channels in"=w885, "auto start"=TRUE, "data"=w880, "error in"=w884) -> ("task out"=w887:refnum<k21>, "error out"=w888:errorcluster)  [unwired: 9 in, 1 out]
    n453 = call <vilib>:"DAQmx Clear Task.vi"("task in"=w904, "error in"=w905) -> ("error out"=w899:errorcluster)  [unwired: 13 in]
    n454 = call <vilib>:"DAQmx Clear Task.vi"("task in"=w887, "error in"=w888) -> ("error out"=w882:errorcluster)  [unwired: 13 in]
    n455 = call <vilib>:"Simple Error Handler.vi"("error in (no error)"=w899) -> ()  [unwired: 4 in, 5 out]
    n456 = call <vilib>:"Simple Error Handler.vi"("error in (no error)"=w882) -> ()  [unwired: 4 in, 5 out]
    n457 = call-poly <vilib>:"DAQmx Create Virtual Channel.vi"("lines"=tag "cDAQ1Mod1/port0/line5", "line grouping"=w870) -> ("task out"=w872:refnum<k21>, "error out"=w871:errorcluster)  [unwired: 12 in]
    n458 = call-poly <vilib>:"DAQmx Create Virtual Channel.vi"("lines"=tag "cDAQ1Mod2/port0/line5", "line grouping"=w862) -> ("task out"=w864:refnum<k21>, "error out"=w863:errorcluster)  [unwired: 12 in]
    n459 = Initialize Array("INLET 1,5 ON/OFF 3", 1 ("dimension size")) -> (w859:bool[])
    n460 = call-poly <vilib>:"DAQmx Write.vi"("task/channels in"=w872, "auto start"=TRUE, "data"=w857, "error in"=w871) -> ("task out"=w874:refnum<k21>, "error out"=w875:errorcluster)  [unwired: 9 in, 1 out]
    n461 = call-poly <vilib>:"DAQmx Write.vi"("task/channels in"=w864, "auto start"=TRUE, "data"=w859, "error in"=w863) -> ("task out"=w866:refnum<k21>, "error out"=w867:errorcluster)  [unwired: 9 in, 1 out]
    n462 = call <vilib>:"DAQmx Clear Task.vi"("task in"=w874, "error in"=w875) -> ("error out"=w869:errorcluster)  [unwired: 13 in]
    n463 = call <vilib>:"DAQmx Clear Task.vi"("task in"=w866, "error in"=w867) -> ("error out"=w861:errorcluster)  [unwired: 13 in]
    n464 = call <vilib>:"Simple Error Handler.vi"("error in (no error)"=w869) -> ()  [unwired: 4 in, 5 out]
    n465 = call <vilib>:"Simple Error Handler.vi"("error in (no error)"=w861) -> ()  [unwired: 4 in, 5 out]
  }
  n466 = Compound Arithmetic op=OR(w1, w2, w3, w16, w15, w14) -> (w17:bool)
  "?" <- w17
  n467 = case shown="True" w17 {
    frame False {
    }
    frame True {
      n468 = call <vilib>:"Beep.vi"("use system alert? (T)"=FALSE, "duration (msec)"=u32 2000, "frequency (Hz)"=u32 15000) -> ()  [unwired: 9 in]
    }
  }
  n469 = control-ref of="PnoData"() -> (w49:refnum<vi>)
  n470 = call <instrlib>:"PDI data xyzaer loop.vi"("Data Ready Refnum"=w49, "FrameCount Ctl Ref"=w59, "error in (no error)"=w69, "xyzaer array\nRefnum"=w58, "Stop Ctl Ref"=w67, "pDev"=w68) -> ("error out"=w56:errorcluster, "Loop Iter"=w60:i32, "dup pDev"=w57:u32)  [unwired: 3 out]
  n471 = local write "Loop Iter"(w60) -> ()
  n472 = local write "Stop 9"(w28) -> ()
  n473 = local write "Stop 12"(w22) -> ()
  n474 = call <instrlib>:"PDI action stopcont.vi"("error in (no error)"=w56, "pDev"=w57) -> ("error out"=w65:errorcluster, "Running"=w70:bool, "dup pDev"=w71:u32)  [unwired: 7 out]
  n475 = local write "Stop 8"(w34) -> ()
  n476 = local write "Stop 7"(w40) -> ()
  n477 = local write "Running"(w70) -> ()
  n478 = case shown="No Error" w56 {
    tunnel: w64 -> [w972 _]
    frame No Error {
      # "Success up to here"
      n479 = call "Elapsed Time"("Set Start Time (s)"=w972) -> ("Present Text"=w974:string, "Elapsed Time Text"=w973:string)  [unwired: 4 in, 13 out]
      n480 = local write "Stop Time Text"(w974) -> ()
      n481 = local write "Elapsed Time Text"(w973) -> ()
    }
    frame Error {
      # "Error somewhere;\nStop Time is irrelevant"
    }
  }
  n482 = while {
    tunnel: w28 -> [_]
    tunnel: w24 -> [w978]
    stop <- w988 stop-if-true
    # "If dT and deadtime have similar values, the identification could evaluate deadtime as zero and this generates proportional gain equal to Inf. This code avoid gain changes in this situations."
    # "Autotuning Loop"
    n483 = local read "Control Output 9"() -> (w990:dbl[])
    n484 = local read "Measurement 9"() -> (w989:dbl[])
    n485 = case shown="\"Internal Model Control\"" "Control 9" {
      tunnel: w990 -> [w999 w1007 w1016 w1025]
      tunnel: w989 -> [w998 w1006 w1015 w1024]
      tunnel: [w997 w1005 w1014 w1023] -> w976
      tunnel: [w996 w1004 w1013 w1022] -> w975
      tunnel: w978 -> [w995 w1003 w1012 w1021]
      tunnel: [w994 w1002 w1011 w1020] -> w977
      tunnel: [w993 w1001 w1010 w1019] -> w980
      tunnel: "Type of controller 9" -> [w992 w1000 w1009 w1018]
      frame "Ziegler-Nichols", Default {
        n486 = call-poly <vilib>:"PID Autotuning Design.vi"("Ziegler-Nichols Speed"="Ziegler-Nichols speed 9", "Type of Controller"=w992, "dt (s)"=w995, "Response signal"=w998, "Stimulus signal"=w999) -> ("PID gains"=w993:T3, "response operating point"=w996:dbl, "stimulus operating point"=w997:dbl, "Plant Parameters"=w994:T5)  [unwired: 3 in]
      }
      frame "Cohen-Coon" {
        n487 = call-poly <vilib>:"PID Autotuning Design.vi"("Type of Controller"=w1000, "dt (s)"=w1003, "Response signal"=w1006, "Stimulus signal"=w1007) -> ("PID gains"=w1001:T3, "response offset"=w1004:dbl, "stimulus offset"=w1005:dbl, "Plant Parameters"=w1002:T5)  [unwired: 4 in]
      }
      frame "Chien-Hrones-Reswick" {
        n488 = call-poly <vilib>:"PID Autotuning Design.vi"("Tuning specifications"="Tuning specifications 9", "Type of Controller"=w1009, "dt (s)"=w1012, "Response signal"=w1015, "Stimulus signal"=w1016) -> ("PID gains"=w1010:T3, "response offset"=w1013:dbl, "stimulus offset"=w1014:dbl, "Plant Parameters"=w1011:T5)  [unwired: 3 in]
      }
      frame "Internal Model Control" {
        n489 = call-poly <vilib>:"PID Autotuning Design.vi"("Desired Time Constant (tau_c)"="Multiplicative factor 9", "Type of Controller"=w1018, "dt (s)"=w1021, "Response signal"=w1024, "Stimulus signal"=w1025) -> ("PID gains"=w1019:T3, "response offset"=w1022:dbl, "stimulus offset"=w1023:dbl, "Plant Parameters"=w1020:T5)  [unwired: 3 in]
      }
    }
    "Identified Plant Parameters 9" <- w977
    "Response operating point 9" <- w975
    "Stimulus operating point 9" <- w976
    n490 = Unbundle(w980) -> ("proportional gain (Kc)"=w983:dbl)  [unwired: 2 out]
    n491 = Equal?(x=w983, y=inf) -> (x = y?=w982:bool)
    n492 = feedback #15() -> (w981:T3)  [unwired: 1 in]
    n493 = Select(t=w981, s=w982, f=w980) -> (s? t:f=w979:T3)
    "Tuned PID gains 9" <- w979
    n494 = feedback-in #15(w979) -> ()
    n495 = case shown="True" "Accept gain 9" {
      tunnel: w979 -> [_ w1026]
      frame False {
      }
      frame True {
        n496 = local write "PID Gains 9"(w1026) -> ()
      }
    }
    n497 = local read "Stop 9"() -> (w988:bool)
  }
  n498 = while {
    tunnel: w22 -> [_]
    tunnel: w18 -> [w1030]
    stop <- w1040 stop-if-true
    # "If dT and deadtime have similar values, the identification could evaluate deadtime as zero and this generates proportional gain equal to Inf. This code avoid gain changes in this situations."
    # "Autotuning Loop"
    n499 = local read "Control Output 12"() -> (w1042:dbl[])
    n500 = local read "Measurement 12"() -> (w1041:dbl[])
    n501 = case shown="\"Ziegler-Nichols\", Default" "Control 12" {
      tunnel: w1042 -> [w1051 w1059 w1068 w1077]
      tunnel: w1041 -> [w1050 w1058 w1067 w1076]
      tunnel: [w1049 w1057 w1066 w1075] -> w1028
      tunnel: [w1048 w1056 w1065 w1074] -> w1029
      tunnel: w1030 -> [w1047 w1055 w1064 w1073]
      tunnel: [w1046 w1054 w1063 w1072] -> w1027
      tunnel: [w1045 w1053 w1062 w1071] -> w1032
      tunnel: "Type of controller 12" -> [w1044 w1052 w1061 w1070]
      frame "Ziegler-Nichols", Default {
        n502 = call-poly <vilib>:"PID Autotuning Design.vi"("Ziegler-Nichols Speed"="Ziegler-Nichols speed 12", "Type of Controller"=w1044, "dt (s)"=w1047, "Response signal"=w1050, "Stimulus signal"=w1051) -> ("PID gains"=w1045:T3, "response operating point"=w1048:dbl, "stimulus operating point"=w1049:dbl, "Plant Parameters"=w1046:T5)  [unwired: 3 in]
      }
      frame "Cohen-Coon" {
        n503 = call-poly <vilib>:"PID Autotuning Design.vi"("Type of Controller"=w1052, "dt (s)"=w1055, "Response signal"=w1058, "Stimulus signal"=w1059) -> ("PID gains"=w1053:T3, "response offset"=w1056:dbl, "stimulus offset"=w1057:dbl, "Plant Parameters"=w1054:T5)  [unwired: 4 in]
      }
      frame "Chien-Hrones-Reswick" {
        n504 = call-poly <vilib>:"PID Autotuning Design.vi"("Tuning specifications"="Tuning specifications 12", "Type of Controller"=w1061, "dt (s)"=w1064, "Response signal"=w1067, "Stimulus signal"=w1068) -> ("PID gains"=w1062:T3, "response offset"=w1065:dbl, "stimulus offset"=w1066:dbl, "Plant Parameters"=w1063:T5)  [unwired: 3 in]
      }
      frame "Internal Model Control" {
        n505 = call-poly <vilib>:"PID Autotuning Design.vi"("Desired Time Constant (tau_c)"="Multiplicative factor 12", "Type of Controller"=w1070, "dt (s)"=w1073, "Response signal"=w1076, "Stimulus signal"=w1077) -> ("PID gains"=w1071:T3, "response offset"=w1074:dbl, "stimulus offset"=w1075:dbl, "Plant Parameters"=w1072:T5)  [unwired: 3 in]
      }
    }
    "Identified Plant Parameters 12" <- w1027
    "Response operating point 12" <- w1029
    "Stimulus operating point 12" <- w1028
    n506 = Unbundle(w1032) -> ("proportional gain (Kc)"=w1035:dbl)  [unwired: 2 out]
    n507 = Equal?(x=w1035, y=inf) -> (x = y?=w1034:bool)
    n508 = feedback #16() -> (w1033:T3)  [unwired: 1 in]
    n509 = Select(t=w1033, s=w1034, f=w1032) -> (s? t:f=w1031:T3)
    "Tuned PID gains 12" <- w1031
    n510 = feedback-in #16(w1031) -> ()
    n511 = case shown="True" "Accept gain 12" {
      tunnel: w1031 -> [_ w1078]
      frame False {
      }
      frame True {
        n512 = local write "PID Gains 12"(w1078) -> ()
      }
    }
    n513 = local read "Stop 12"() -> (w1040:bool)
  }
  n514 = while {
    tunnel: w34 -> [_]
    tunnel: w30 -> [w1082]
    stop <- w1092 stop-if-true
    # "If dT and deadtime have similar values, the identification could evaluate deadtime as zero and this generates proportional gain equal to Inf. This code avoid gain changes in this situations."
    # "Autotuning Loop"
    n515 = local read "Control Output 8"() -> (w1094:dbl[])
    n516 = local read "Measurement 8"() -> (w1093:dbl[])
    n517 = case shown="\"Chien-Hrones-Reswick\"" "Control 8" {
      tunnel: w1094 -> [w1103 w1111 w1120 w1129]
      tunnel: w1093 -> [w1102 w1110 w1119 w1128]
      tunnel: [w1101 w1109 w1118 w1127] -> w1081
      tunnel: [w1100 w1108 w1117 w1126] -> w1080
      tunnel: w1082 -> [w1099 w1107 w1116 w1125]
      tunnel: [w1098 w1106 w1115 w1124] -> w1079
      tunnel: [w1097 w1105 w1114 w1123] -> w1084
      tunnel: "Type of controller 8" -> [w1096 w1104 w1113 w1122]
      frame "Ziegler-Nichols", Default {
        n518 = call-poly <vilib>:"PID Autotuning Design.vi"("Ziegler-Nichols Speed"="Ziegler-Nichols speed 8", "Type of Controller"=w1096, "dt (s)"=w1099, "Response signal"=w1102, "Stimulus signal"=w1103) -> ("PID gains"=w1097:T3, "response operating point"=w1100:dbl, "stimulus operating point"=w1101:dbl, "Plant Parameters"=w1098:T5)  [unwired: 3 in]
      }
      frame "Cohen-Coon" {
        n519 = call-poly <vilib>:"PID Autotuning Design.vi"("Type of Controller"=w1104, "dt (s)"=w1107, "Response signal"=w1110, "Stimulus signal"=w1111) -> ("PID gains"=w1105:T3, "response offset"=w1108:dbl, "stimulus offset"=w1109:dbl, "Plant Parameters"=w1106:T5)  [unwired: 4 in]
      }
      frame "Chien-Hrones-Reswick" {
        n520 = call-poly <vilib>:"PID Autotuning Design.vi"("Tuning specifications"="Tuning specifications 8", "Type of Controller"=w1113, "dt (s)"=w1116, "Response signal"=w1119, "Stimulus signal"=w1120) -> ("PID gains"=w1114:T3, "response offset"=w1117:dbl, "stimulus offset"=w1118:dbl, "Plant Parameters"=w1115:T5)  [unwired: 3 in]
      }
      frame "Internal Model Control" {
        n521 = call-poly <vilib>:"PID Autotuning Design.vi"("Desired Time Constant (tau_c)"="Multiplicative factor 8", "Type of Controller"=w1122, "dt (s)"=w1125, "Response signal"=w1128, "Stimulus signal"=w1129) -> ("PID gains"=w1123:T3, "response offset"=w1126:dbl, "stimulus offset"=w1127:dbl, "Plant Parameters"=w1124:T5)  [unwired: 3 in]
      }
    }
    "Stimulus operating point 8" <- w1081
    "Response operating point 8" <- w1080
    "Identified Plant Parameters 8" <- w1079
    n522 = Unbundle(w1084) -> ("proportional gain (Kc)"=w1087:dbl)  [unwired: 2 out]
    n523 = Equal?(x=w1087, y=inf) -> (x = y?=w1086:bool)
    n524 = feedback #17() -> (w1085:T3)  [unwired: 1 in]
    n525 = Select(t=w1085, s=w1086, f=w1084) -> (s? t:f=w1083:T3)
    "Tuned PID gains 8" <- w1083
    n526 = feedback-in #17(w1083) -> ()
    n527 = case shown="True" "Accept gain 8" {
      tunnel: w1083 -> [_ w1130]
      frame False {
      }
      frame True {
        n528 = local write "PID Gains 8"(w1130) -> ()
      }
    }
    n529 = local read "Stop 8"() -> (w1092:bool)
  }
  n530 = while {
    tunnel: w40 -> [_]
    tunnel: w36 -> [w1134]
    stop <- w1144 stop-if-true
    # "If dT and deadtime have similar values, the identification could evaluate deadtime as zero and this generates proportional gain equal to Inf. This code avoid gain changes in this situations."
    # "Autotuning Loop"
    n531 = local read "Control Output 7"() -> (w1146:dbl[])
    n532 = local read "Measurement 7"() -> (w1145:dbl[])
    n533 = case shown="\"Chien-Hrones-Reswick\"" "Control 7" {
      tunnel: w1146 -> [w1155 w1163 w1172 w1181]
      tunnel: w1145 -> [w1154 w1162 w1171 w1180]
      tunnel: [w1153 w1161 w1170 w1179] -> w1133
      tunnel: [w1152 w1160 w1169 w1178] -> w1132
      tunnel: w1134 -> [w1151 w1159 w1168 w1177]
      tunnel: [w1150 w1158 w1167 w1176] -> w1131
      tunnel: [w1149 w1157 w1166 w1175] -> w1136
      tunnel: "Type of controller 7" -> [w1148 w1156 w1165 w1174]
      frame "Ziegler-Nichols", Default {
        n534 = call-poly <vilib>:"PID Autotuning Design.vi"("Ziegler-Nichols Speed"="Ziegler-Nichols speed 7", "Type of Controller"=w1148, "dt (s)"=w1151, "Response signal"=w1154, "Stimulus signal"=w1155) -> ("PID gains"=w1149:T3, "response operating point"=w1152:dbl, "stimulus operating point"=w1153:dbl, "Plant Parameters"=w1150:T5)  [unwired: 3 in]
      }
      frame "Cohen-Coon" {
        n535 = call-poly <vilib>:"PID Autotuning Design.vi"("Type of Controller"=w1156, "dt (s)"=w1159, "Response signal"=w1162, "Stimulus signal"=w1163) -> ("PID gains"=w1157:T3, "response offset"=w1160:dbl, "stimulus offset"=w1161:dbl, "Plant Parameters"=w1158:T5)  [unwired: 4 in]
      }
      frame "Chien-Hrones-Reswick" {
        n536 = call-poly <vilib>:"PID Autotuning Design.vi"("Tuning specifications"="Tuning specifications 7", "Type of Controller"=w1165, "dt (s)"=w1168, "Response signal"=w1171, "Stimulus signal"=w1172) -> ("PID gains"=w1166:T3, "response offset"=w1169:dbl, "stimulus offset"=w1170:dbl, "Plant Parameters"=w1167:T5)  [unwired: 3 in]
      }
      frame "Internal Model Control" {
        n537 = call-poly <vilib>:"PID Autotuning Design.vi"("Desired Time Constant (tau_c)"="Multiplicative factor 7", "Type of Controller"=w1174, "dt (s)"=w1177, "Response signal"=w1180, "Stimulus signal"=w1181) -> ("PID gains"=w1175:T3, "response offset"=w1178:dbl, "stimulus offset"=w1179:dbl, "Plant Parameters"=w1176:T5)  [unwired: 3 in]
      }
    }
    "Stimulus operating point 7" <- w1133
    "Response operating point 7" <- w1132
    "Identified Plant Parameters 7" <- w1131
    n538 = Unbundle(w1136) -> ("proportional gain (Kc)"=w1139:dbl)  [unwired: 2 out]
    n539 = Equal?(x=w1139, y=inf) -> (x = y?=w1138:bool)
    n540 = feedback #18() -> (w1137:T3)  [unwired: 1 in]
    n541 = Select(t=w1137, s=w1138, f=w1136) -> (s? t:f=w1135:T3)
    "Tuned PID gains 7" <- w1135
    n542 = feedback-in #18(w1135) -> ()
    n543 = case shown="True" "Accept gain 7" {
      tunnel: w1135 -> [_ w1182]
      frame False {
      }
      frame True {
        n544 = local write "PID Gains 7"(w1182) -> ()
      }
    }
    n545 = local read "Stop 7"() -> (w1144:bool)
  }
  n546 = call <instrlib>:"PDI close.vi"("error in (no error)"=w65, "pDev"=w71) -> ("error out"=→"error out":errorcluster, "connected"=w66:bool)  [unwired: 8 out]
  n547 = local write "Connected"(w66) -> ()
